vi "Main.vi"() -> ()   [LabVIEW 2020]
uses:
  <vilib>/Modbus/master/Modbus Master.lvclass
  ctl/StationAction.ctl
  <vilib>/Analysis/baseanly.llb/Mean (DBL).vi
  <vilib>/Modbus/master/Create Master Instance (TCP).vi
  <vilib>/Utility/file.llb/Read Delimited Spreadsheet (string).vi
  <vilib>/Analysis/NI_AALBase.lvlib
panel:
  out "原始表格":string[][](table)
  in  "LabVIEW._Application 6":refnum<k7>
  out "权限out":i32
  out "用户名out":string
  out "用户信息out":string[][](array[string]) caption="所有行"
  out "error out 3":errorcluster caption="错误输出"
  out "error out 2":errorcluster caption="错误输出"
  out "error out":errorcluster caption="错误输出"
  out "PLC状态显示":string
  out "PLC_Hd":refnum<class "Modbus Master.lvclass"> caption="TCP主设备实例"
  in  "确定按钮 2":bool
  in  "确定按钮":bool
  in  "LabVIEW._Application 5":refnum<k7>
  out "Cpk原始数据":string[][](array[string])
  in  "Btn_Exit":bool
  in  "选项卡控件":enum32{"工位1", "工位2", "数据分析"}(tab)
  in  "启动信号":u16
  in  "数组":string[](array[string])
  out "工位1_实时压力_Ind":string caption="实时压力"
  out "工位1_数据图表显示":cluster{i32[], dbl[]}[](graph)
  out "工位1_产品型号":string caption="产品型号"
  in  "数组 2":string[](array[string])
  in  "启动信号 2":u16
  out "工位2_产品型号":string caption="产品型号"
  out "工位2_实时压力_Ind":string caption="实时压力"
  out "工位2_数据图表显示":cluster{i32[], dbl[]}[](graph)
  in  "Btn_导出数据":bool
  in  "Btn_保存报告":bool
  out "Cpk":dbl format="%.2f"
  out "均值":dbl
  out "下限值":dbl
  out "上限值":dbl
  out "最小值":dbl
  out "最大值":dbl
  in  "Btn_分析计算":bool
  in  "终止行":u32=10 min=2 step=1
  in  "Cpk保存路径":path
  out "表格控件":string[][](table)
  in  "起始行":u32=1 min=1 step=1
  in  "工位号":enum16{"工位1", "工位2"}(ring)
  out "paramVals":variant
  in  "LabVIEW._Application 4":refnum<k7>
  out "工位1_数据表显示":string[][](table)
  out "bExit?":bool
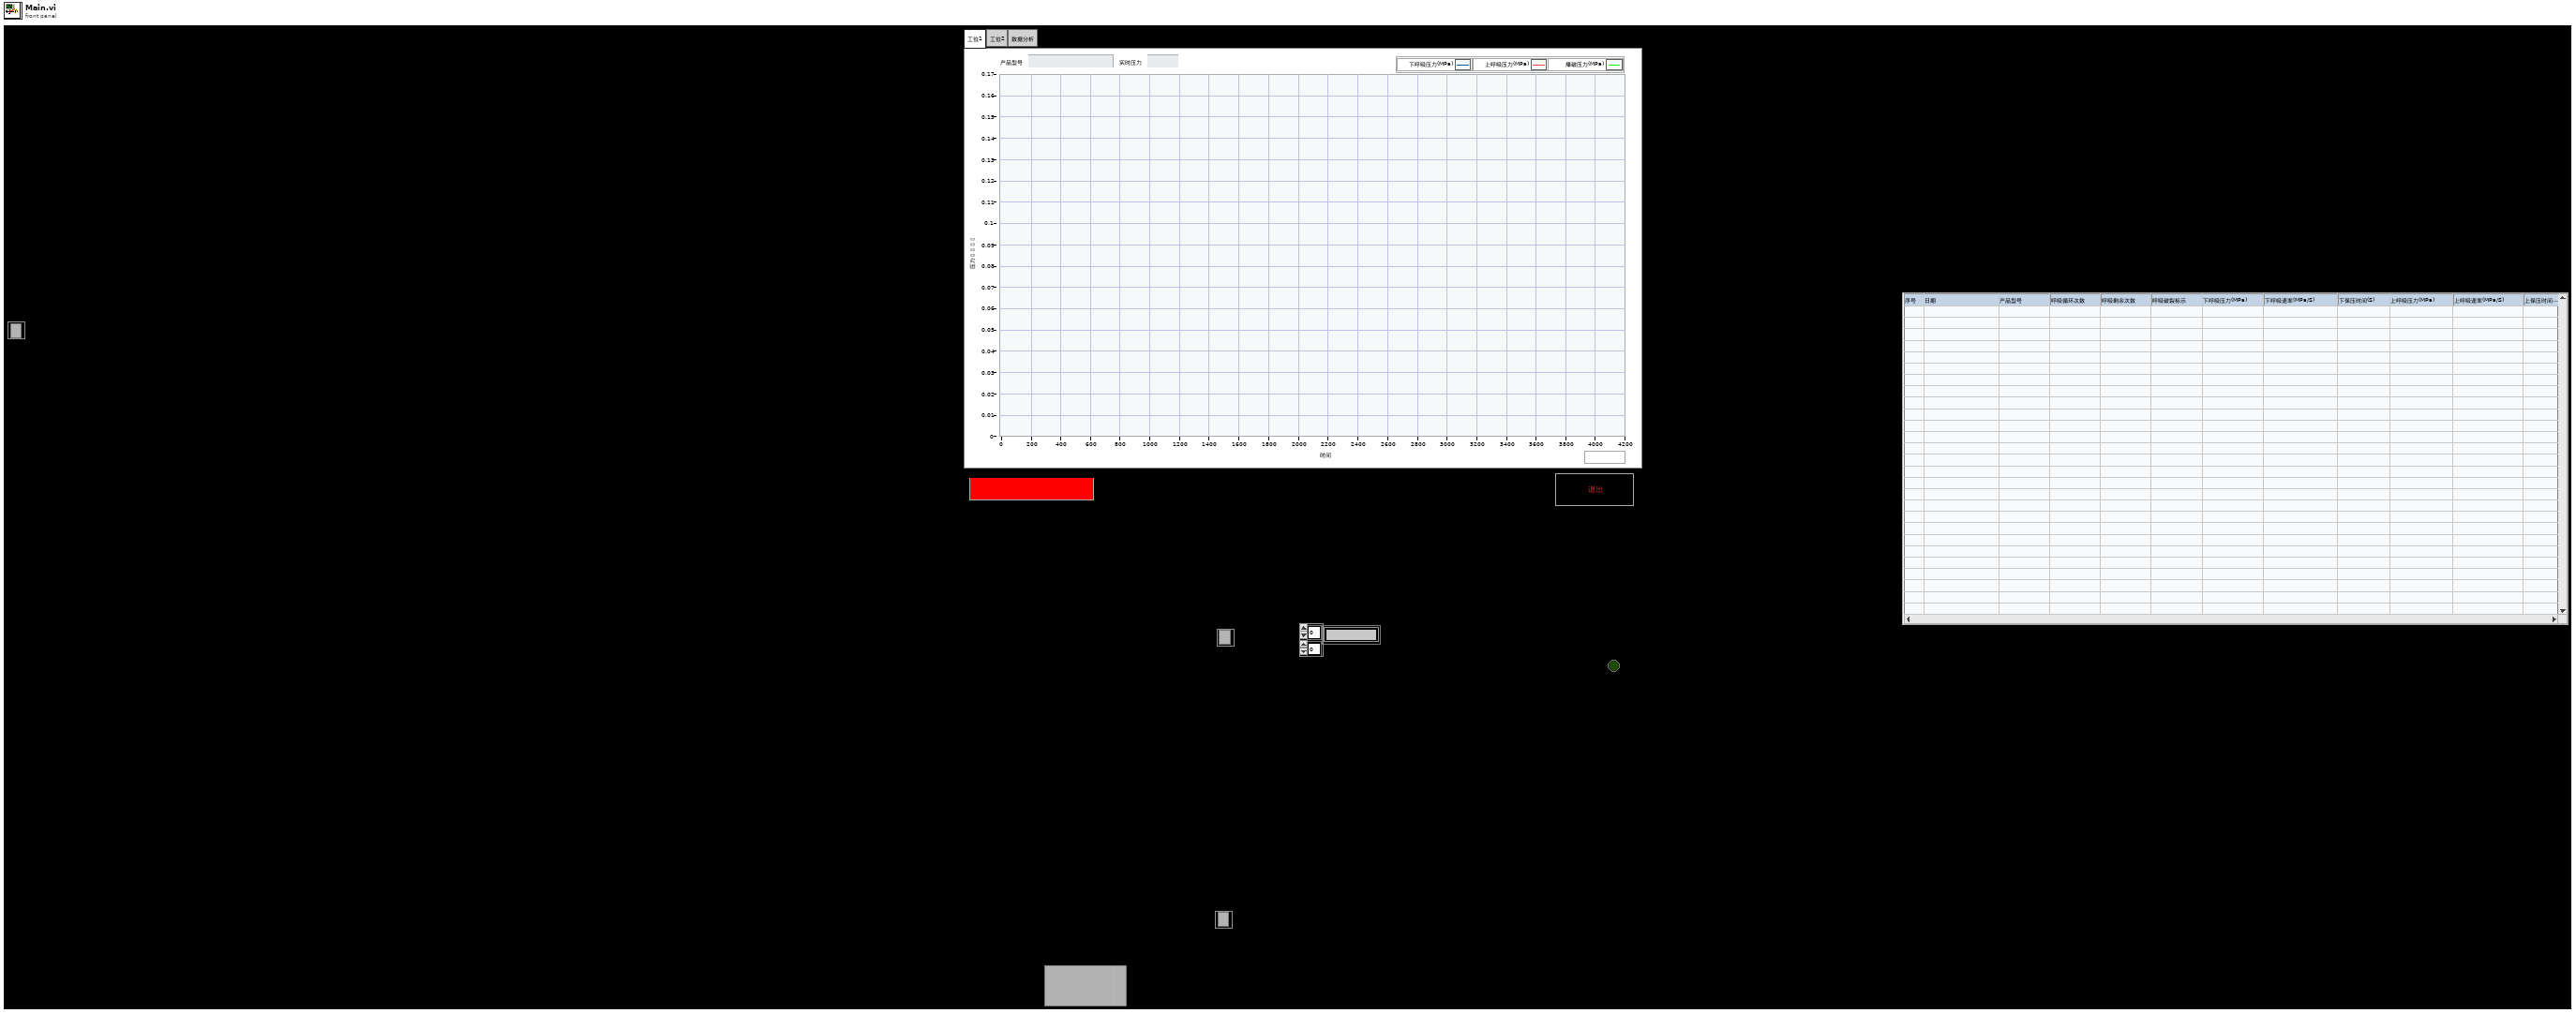
[diagram p1: front panel]
types:
  T1 = typedef "StationAction.ctl" = enum16{"Init", "Monitor", "Done", "Exit"}
  T2 = enum8{"Enabled", "Disabled", "Disabled and Grayed Out"}
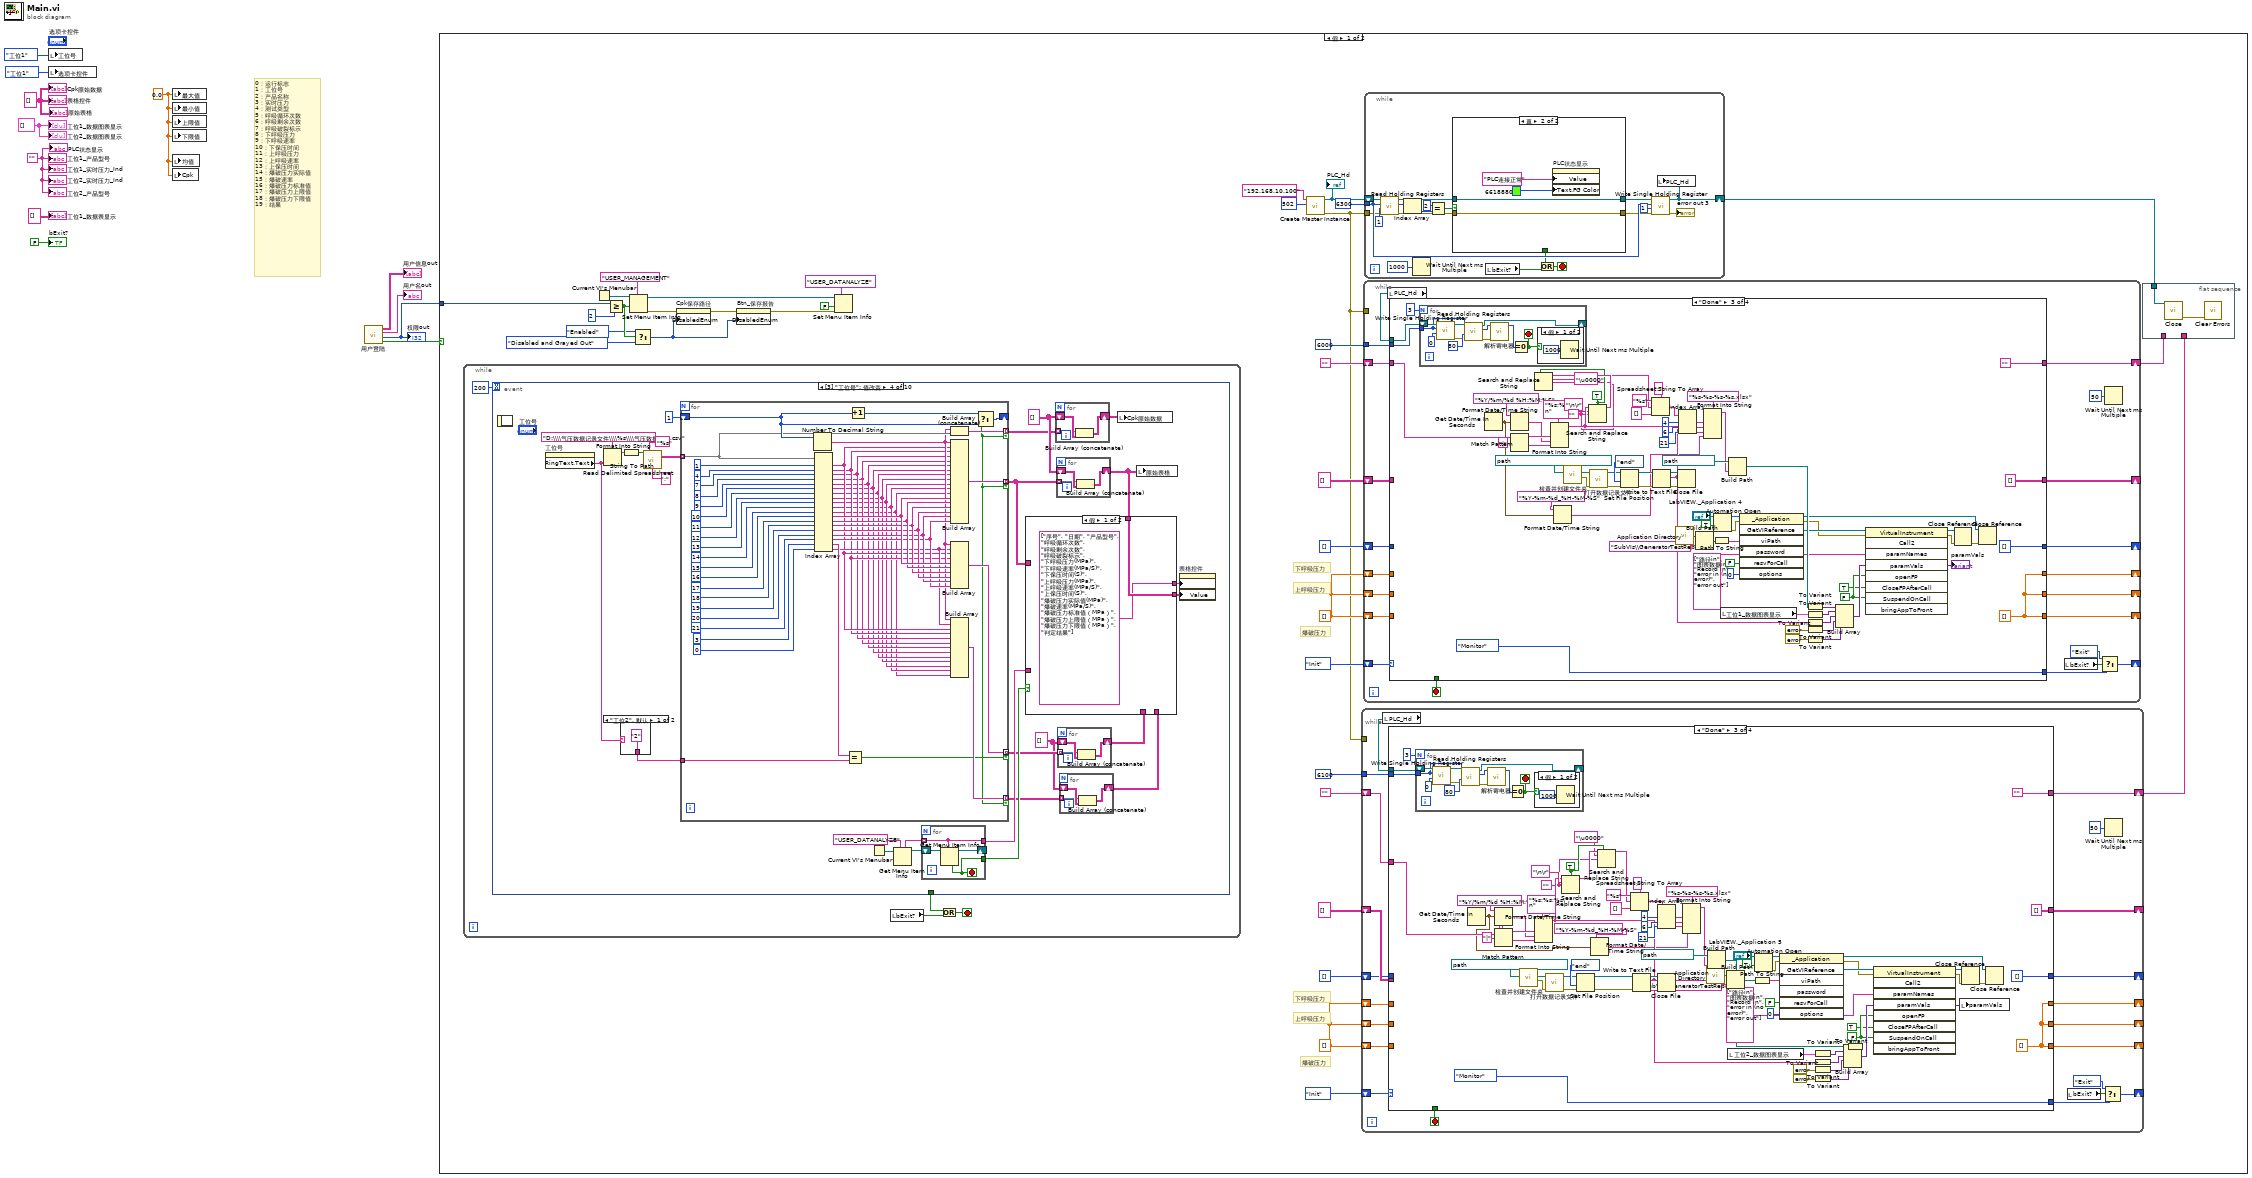
[diagram p0: block diagram]
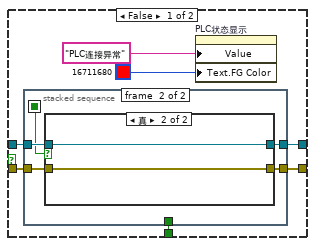
[diagram p2: hidden frame]
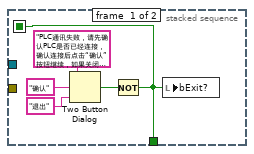
[diagram p3: hidden frame]
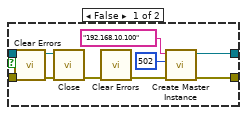
[diagram p4: hidden frame]
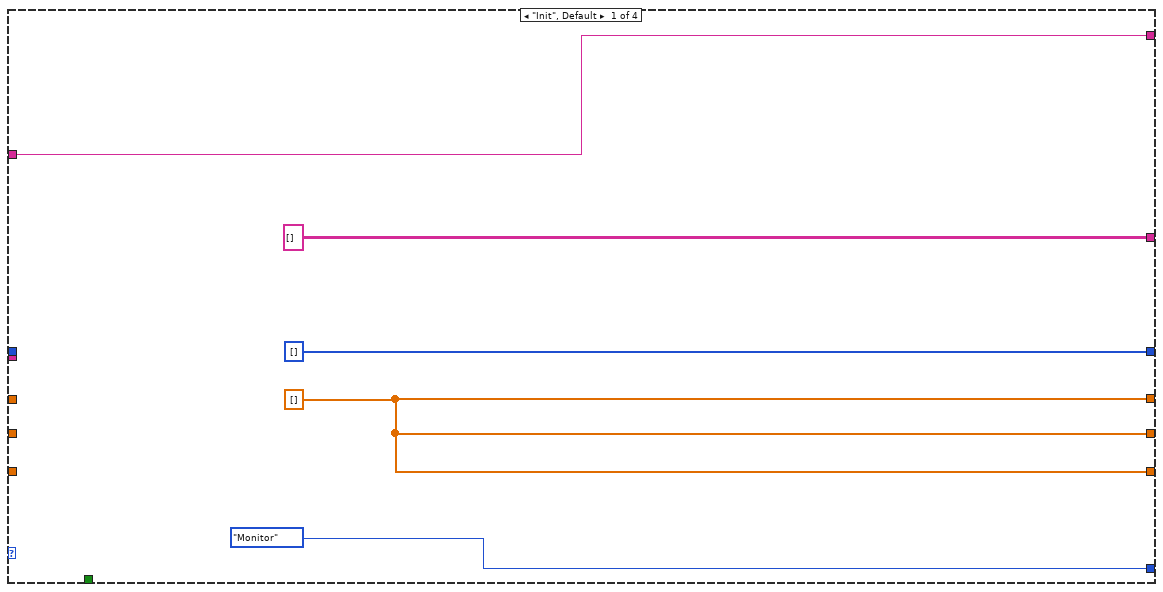
[diagram p5: hidden frame]
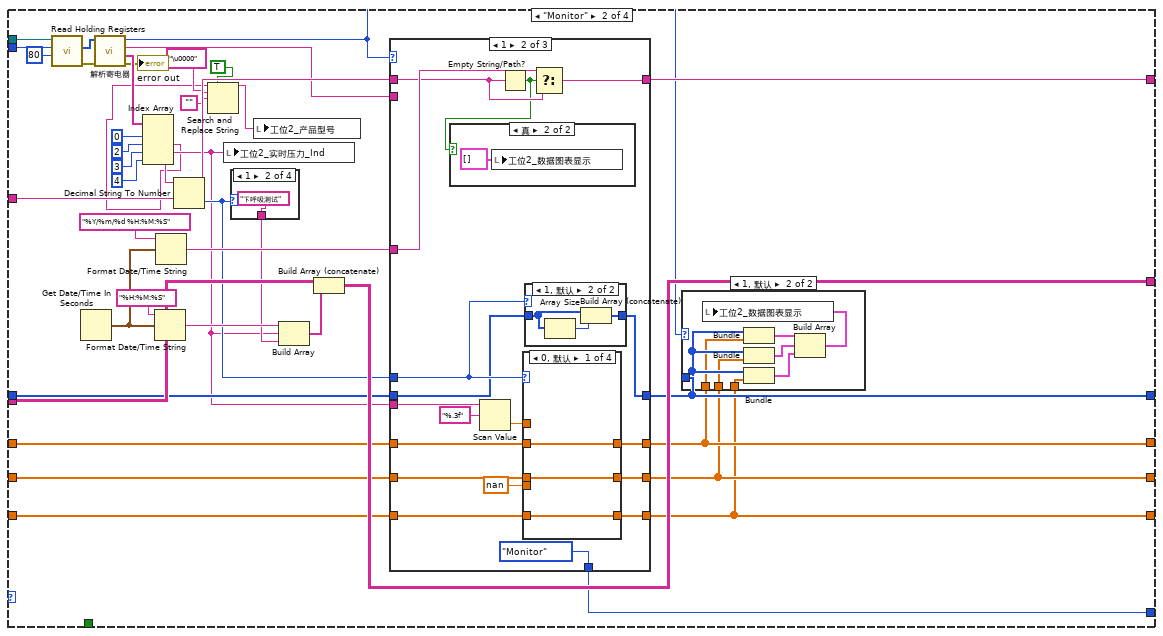
[diagram p6: hidden frame]
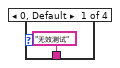
[diagram p8: hidden frame]
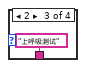
[diagram p9: hidden frame]
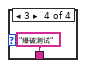
[diagram p10: hidden frame]
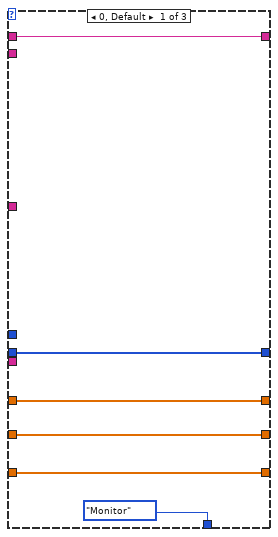
[diagram p11: hidden frame]
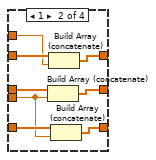
[diagram p14: hidden frame]
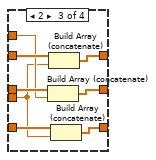
[diagram p15: hidden frame]
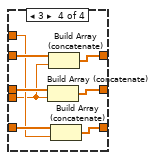
[diagram p16: hidden frame]
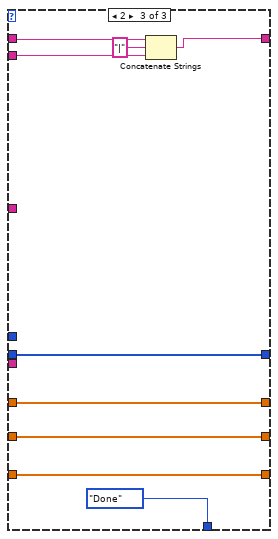
[diagram p17: hidden frame]
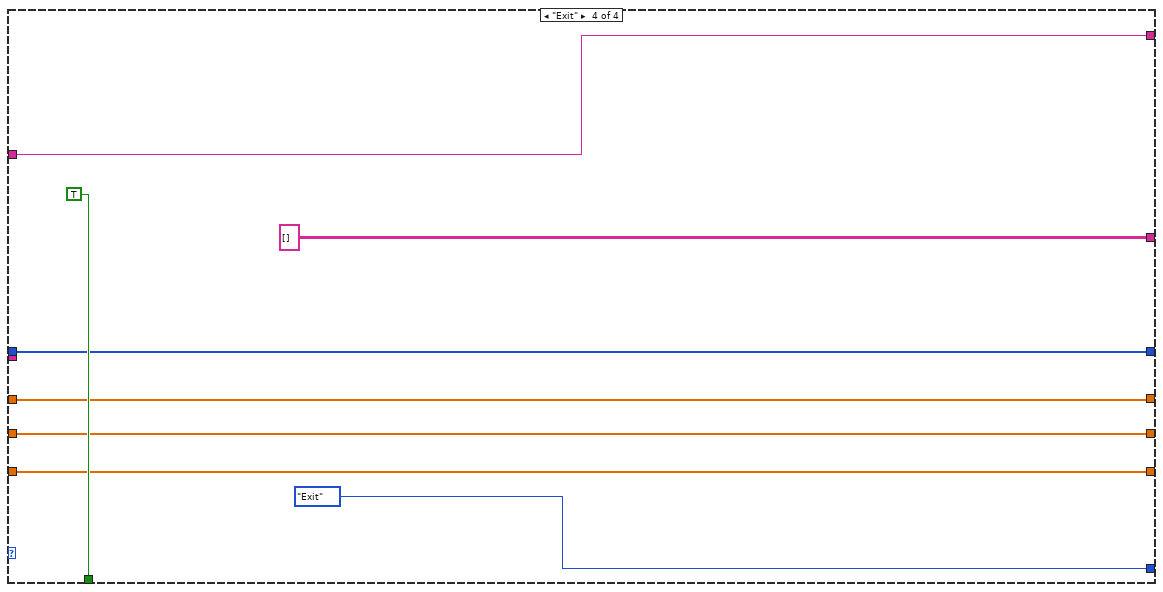
[diagram p19: hidden frame]
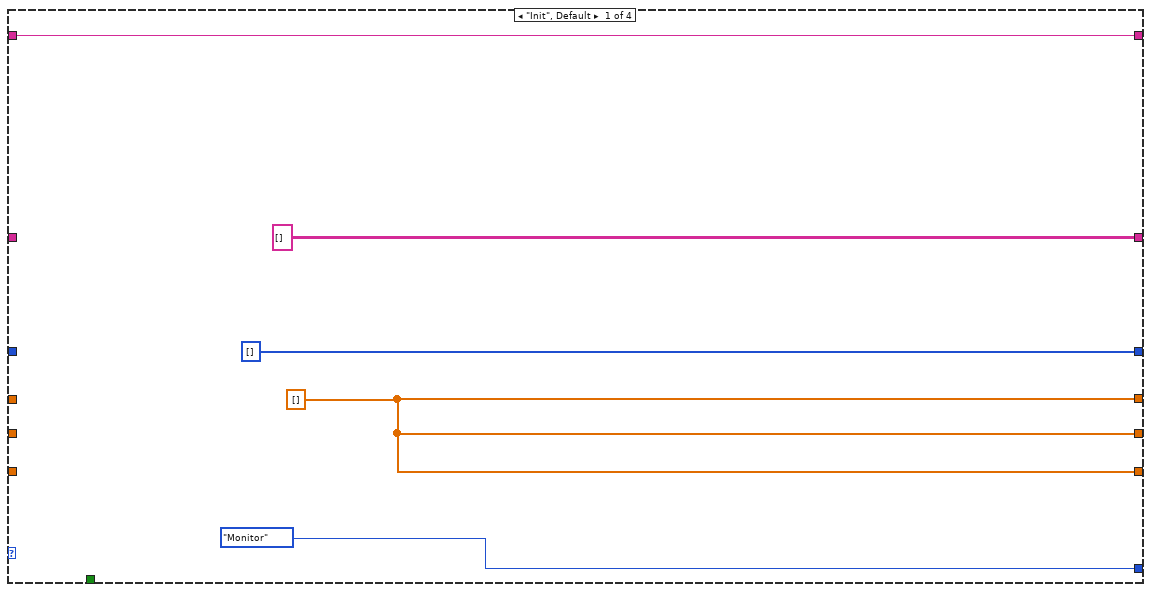
[diagram p20: hidden frame]
diagram:
  w7 = 0.0 ("最大值")
  w1 = string[][] [] ("表格控件")
  w8 = cluster{i32[], dbl[]}[] [] ("添加的数组")
  w6 = ""
  # "0：运行标志\n1：工位号\n2：产品名称\n3：实时压力\n4：测试类型\n5：呼吸循环次数\n6：呼吸剩余次数\n7：呼吸破裂标示\n8：下呼吸压力\n9：下呼吸速率\n10：下保压时间\n11：上呼吸压力\n12：上呼吸速率\n13：上保压时间\n14：爆破压力实际值\n15：爆破速率\n16：爆破压力标准值\n17：爆破压力上限值\n18：爆破压力下限值\n19：结果"
  n1 = local write "工位号"(enum16{"工位1", "工位2"}."工位1" ("工位号")) -> ()
  n2 = local write "选项卡控件"(enum32{"工位1", "工位2", "数据分析"}."工位1" ("选项卡控件")) -> ()
  n3 = local write "最大值"(w7) -> ()
  n4 = local write "最小值"(w7) -> ()
  n5 = local write "上限值"(w7) -> ()
  n6 = local write "下限值"(w7) -> ()
  n7 = local write "均值"(w7) -> ()
  n8 = local write "Cpk"(w7) -> ()
  n9 = call "用户登陆.vi"() -> ("退出"=w5:bool, "权限out"=w2:i32, "用户名out"=→"用户名out":string, "用户信息out"=→"用户信息out":string[][])  [unwired: 8 in]
  "权限out" <- w2
  n10 = case shown="假" w5 {
    tunnel: w2 -> [w44 _]
    frame False {
      w27 = dbl[] []
      w28 = dbl[] []
      # "爆破压力"
      # "上呼吸压力"
      # "下呼吸压力"
      # "爆破压力"
      # "上呼吸压力"
      # "下呼吸压力"
      n11 = while {
        stop <- w585 stop-if-true
        n12 = event shown="[3] \"工位号\": 值改变" {
          selector: _ -> [_ _ _ _ _ _ _ _ _ _]
          dyn-events: _ -> [_ _ _ _ _ _ _ _ _ _]
          timeout: 200 -> [_ _ _ _ _ _ _ _ _ _]
          tunnel: [_ "Btn_Exit" _ _ _ _ _ _ _ _] -> w586
          event Timeout {
            n13 = event-data() -> ()  [unwired: 1 in, 3 out]
          }
          event "Btn_Exit": Value Change {
            n14 = event-data() -> ()  [unwired: 1 in, 1 out]
            n15 = local write "bExit?"("Btn_Exit") -> ()
          }
          event "Btn_分析计算": Value Change {
            n16 = event-data() -> ()  [unwired: 1 in, 1 out]
            n17 = local read "原始表格"() -> (w591:string[][])
            n18 = Subtract(x="终止行", y="起始行") -> (x-y=w593:u32)
            n19 = Less Than 0?(x=w593) -> (x < 0?=w594:bool)
            n20 = Empty Array?(array=w591) -> (empty?=w592:bool)
            n21 = Increment(x=w593) -> (x+1=w589:u32)
            n22 = case shown="假" w592 {
              tunnel: w594 -> [w599 _]
              tunnel: w589 -> [w598 _]
              tunnel: w591 -> [w597 _]
              tunnel: "起始行" -> [w596 _]
              frame False {
                n23 = case shown="假" w599 {
                  tunnel: w598 -> [w601 _]
                  tunnel: w597 -> [w604 _]
                  tunnel: w596 -> [w603 _]
                  frame False {
                    n24 = Greater Or Equal?(x=w601, y=2 ("禁用的索引 (列)")) -> (x >= y?=w602:bool)
                    n25 = case shown="真" w602 {
                      tunnel: w604 -> [_ w634]
                      tunnel: w601 -> [_ w606]
                      tunnel: w603 -> [_ w608]
                      frame False {
                        n26 = One Button Dialog(message="选择数据的数量至少需要2个" ("消息")) -> ()  [unwired: 1 in, 1 out]
                      }
                      frame True {
                        w626 = 0 ("禁用的索引 (列)")
                        n27 = Decrement(x=w608) -> (x-1=w607:u32)
                        n28 = Array Subset(array=w634, index (row)=w607, length (row)=w606) -> (w633:string[][])  [unwired: 2 in]
                        n29 = Fract/Exp String To Number(string=w633) -> (number=w632:dbl[][])  [unwired: 3 in, 1 out]
                        n30 = Index Array(array=w632, index (col) #1=12 ("禁用的索引 (列)"), index (row) #2=w626, index (col) #2=14 ("禁用的索引 (列)"), index (row) #3=w626, index (col) #3=15 ("禁用的索引 (列)"), index (row) #4=w626, index (col) #4=16 ("禁用的索引 (列)")) -> (element #1=w624:dbl[], element #2=w623:dbl, element #3=w620:dbl, element #4=w619:dbl)  [unwired: 1 in]
                        "上限值" <- w620
                        "下限值" <- w619
                        n31 = Array Max & Min(array=w624) -> (max value=→"最大值":dbl, min value=→"最小值":dbl)  [unwired: 2 out]
                        n32 = call-poly <vilib>:"Mean.vi"("X"=w624) -> ("mean"=w622:dbl)  [unwired: 1 out]
                        "均值" <- w622
                        n33 = call <vilib>:"Std Deviation and Variance.vi"("X"=w624) -> ("standard deviation"=w615:dbl)  [unwired: 1 in, 2 out]
                        n34 = Subtract(x=w622, y=w623) -> (x-y=w621:dbl)
                        n35 = Subtract(x=w620, y=w619) -> (x-y=w613:dbl)
                        n36 = Absolute Value(x=w621) -> (abs(x)=w618:dbl)
                        n37 = Multiply(x=w615, y=3.0) -> (x*y=w617:dbl)
                        n38 = Multiply(x=w615, y=6.0) -> (x*y=w612:dbl)
                        n39 = Divide(x=w618, y=w617) -> (x/y=w610:dbl)
                        n40 = Divide(x=w613, y=w612) -> (x/y=w611:dbl)
                        n41 = Subtract(x=w611, y=w610) -> (x-y=→"Cpk":dbl)
                      }
                    }
                  }
                  frame True {
                    n42 = One Button Dialog(message="终止行必须大于起始行" ("消息")) -> ()  [unwired: 1 in, 1 out]
                  }
                }
              }
              frame True {
                n43 = One Button Dialog(message="参与计算Cpk的数据不可以为空" ("消息")) -> ()  [unwired: 1 in, 1 out]
              }
            }
          }
          event "工位号": Value Change {
            w639 = string[][] []
            w654 = string[][] []
            n44 = event-data() -> ()  [unwired: 1 in, 1 out]
            n45 = property on="工位号" class="Enum (严格)"() -> ("RingText.Text"=w657:string)  [unwired: 2 in, 2 out]
            n46 = Format Into String(format string="D:\\\\气压数据记录文件\\\\%s\\\\气压数据记录.csv" ("格式字符串"), w657) -> (resulting string=w661:string)  [unwired: 2 in, 1 out]
            n47 = case shown="\"工位2\", 默认" w657 {
              tunnel: ["2" ("delimiter (\\t)") "1" ("delimiter (\\t)")] -> w656
              frame "工位2", Default {
              }
              frame "工位1" {
              }
            }
            n48 = String To Path(string=w661) -> (path=w660:path)
            n49 = call-poly <vilib>:"Read Delimited Spreadsheet.vi"("file path (dialog if empty)"=w660, "format (%s)"="%s", "delimiter (\\t)"=";" ("delimiter (\\t)")) -> ("all rows"=w658:string[][])  [unwired: 7 in, 5 out]
            n50 = for {
              tunnel: w658 -> [w721] mode=indexing
              tunnel: [w728] -> w645 mode=indexing if=w697
              tunnel: w656 -> [w727]
              tunnel: [w720] -> w653 mode=indexing if=w697
              shift-right: [w723] -> _
              shift-left: 1 -> [w722]
              tunnel: [w712] -> w641 mode=indexing if=w697
              tunnel: [w698] -> w638 mode=indexing if=w697
              n51 = Number To Decimal String(number=w722) -> (decimal integer string=w711:string)  [unwired: 1 in]
              n52 = Index Array(array=w721, index #1=1 ("索引"), index #2=4 ("索引"), index #3=7 ("索引"), index #4=8 ("索引"), index #5=9 ("索引"), index #6=10 ("索引"), index #7=11 ("索引"), index #8=12 ("索引"), index #9=13 ("索引"), index #10=14 ("索引"), index #11=15 ("索引"), index #12=16 ("索引"), index #13=17 ("索引"), index #14=18 ("索引"), index #15=19 ("索引"), index #16=20 ("索引"), index #17=21 ("索引"), index #18=3 ("索引"), index #19=0 ("索引")) -> (element #1=w709:string, element #2=w708:string, element #3=w707:string, element #4=w706:string, element #5=w705:string, element #6=w704:string, element #7=w703:string, element #8=w702:string, element #9=w701:string, element #10=w700:string, element #11=w699:string, element #12=w718:string, element #13=w717:string, element #14=w716:string, element #15=w715:string, element #16=w714:string, element #17=w713:string, element #18=w725:string, element #19=w710:string)
              n53 = Equal?(x=w725, y=w727) -> (x = y?=w697:bool)
              n54 = Increment(x=w722) -> (x+1=w724:i32)
              n55 = Build Array (concatenate)(w711, w721) -> (w720:string[])
              n56 = Build Array(w711, w709, w708, w707, w706, w705, w704, w703, w702, w701, w700, w699, w718, w717, w716, w715, w714, w713) -> (w728:string[])
              n57 = Build Array(w711, w710, w709, w708, w718, w717, w716, w715, w714, w713) -> (w712:string[])
              n58 = Build Array(w711, w710, w709, w708, w707, w706, w705, w704, w703, w702, w701, w700, w699) -> (w698:string[])
              n59 = Select(t=w724, s=w697, f=w722) -> (s? t:f=w723:i32)
            }
            n60 = Current VI's Menubar() -> (w651:refnum<k9>)
            n61 = Get Menu Item Info(7:"USER_DATANALYZE" ("项标识符"), 11:w651) -> (3:w648:refnum<k9>, 5:w649:string[])  [unwired: 1 in, 5 out]
            n62 = for {
              tunnel: w649 -> [w686] mode=indexing
              shift-right: [w687] -> _
              shift-left: w648 -> [w688]
              tunnel: [w686] -> w646
              tunnel: [w685] -> w647
              stop <- w685 stop-if-true
              n63 = Get Menu Item Info(7:w686, 11:w688) -> (3:w687:refnum<k9>, 4:w685:bool)  [unwired: 1 in, 5 out]
            }
            n64 = for {
              shift-right: [w693] -> w652
              shift-left: w654 -> [w694]
              tunnel: w653 -> [w692] mode=indexing
              n65 = Build Array (concatenate)(w692, w694) -> (w693:string[][])
            }
            n66 = for {
              shift-right: [w690] -> w644
              shift-left: w654 -> [w691]
              tunnel: w645 -> [w689] mode=indexing
              n67 = Build Array (concatenate)(w689, w691) -> (w690:string[][])
            }
            n68 = for {
              shift-right: [w668] -> w640
              shift-left: w639 -> [w669]
              tunnel: w641 -> [w667] mode=indexing
              n69 = Build Array (concatenate)(w667, w669) -> (w668:string[][])
            }
            n70 = for {
              shift-right: [w665] -> w637
              shift-left: w639 -> [w666]
              tunnel: w638 -> [w664] mode=indexing
              n71 = Build Array (concatenate)(w664, w666) -> (w665:string[][])
            }
            n72 = case shown="假" w647 {
              tunnel: w646 -> [_ w677]
              tunnel: w645 -> [_ w678]
              tunnel: [w671 w675] -> w643
              tunnel: w644 -> [w671 w676]
              tunnel: [string[] ["序号", "日期", "产品型号", "呼吸循环次数", "呼吸剩余次数", "呼吸破裂标示", "下呼吸压力(MPa)", "下呼吸速率(MPa/S)", "下保压时间(S)", "上呼吸压力(MPa)", "上呼吸速率(MPa/S)", "上保压时间(S)", "爆破压力实际值(MPa)", "爆破速率(MPa/S)", "爆破压力标准值（MPa）", "爆破压力上限值（MPa）", "爆破压力下限值（MPa）", "判定结果"] w674] -> w642
              tunnel: w640 -> [_ w673]
              tunnel: w637 -> [_ w672]
              frame False {
              }
              frame True {
                n73 = case shown="\"假\", 默认" w677 {
                  tunnel: w678 -> [_ _ _]
                  tunnel: w676 -> [w680 _ _]
                  tunnel: [w680 w681 w683] -> w675
                  tunnel: [string[] ["序号", "日期", "产品型号", "呼吸循环次数", "呼吸剩余次数", "呼吸破裂标示", "下呼吸压力(MPa)", "下呼吸速率(MPa/S)", "下保压时间(S)", "上呼吸压力(MPa)", "上呼吸速率(MPa/S)", "上保压时间(S)", "爆破压力实际值(MPa)", "爆破速率(MPa/S)", "爆破压力标准值（MPa）", "爆破压力上限值（MPa）", "爆破压力下限值（MPa）", "判定结果"] w682 w684] -> w674
                  tunnel: w673 -> [_ w681 _]
                  tunnel: w672 -> [_ _ w683]
                  frame "假", Default {
                  }
                  frame "USER_BLASTING_REC" {
                    w682 = string[] ["序号", "开始时间", "结束时间", "产品型号", "爆破压力实际值(MPa)", "爆破速率(MPa/S)", "爆破压力标准值（MPa）", "爆破压力上限值（MPa）", "爆破压力下限值（MPa）", "判定结果"]  # 爆破记录
                  }
                  frame "USER_BREATHE_REC" {
                    w684 = string[] ["序号", "开始时间", "结束时间", "产品型号", "呼吸循环次数", "呼吸剩余次数", "呼吸破裂标示", "下呼吸压力(MPa)", "下呼吸速率(MPa/S)", "下保压时间(S)", "上呼吸压力(MPa)", "上呼吸速率(MPa/S)", "上保压时间(S)"]  # 呼吸记录
                  }
                }
              }
            }
            n74 = local write "Cpk原始数据"(w652) -> ()
            n75 = local write "原始表格"(w644) -> ()
            n76 = property on="表格控件" class="Tbl (严格)"("Column Headers[]"=w642, "Value"=w643) -> ()  [unwired: 2 in, 2 out]
          }
          event "选项卡控件": Value Change {
            # "0：开始时间\n1：结束时间\n2：运行标志\n3：工位号\n4：产品名称\n5：实时压力\n6：测试类型\n7：呼吸循环次数\n8：呼吸剩余次数\n9：呼吸破裂标示\n10：下呼吸压力\n11：下呼吸速率\n12：下保压时间\n13：上呼吸压力\n14：上呼吸速率\n15：上保压时间\n16：爆破压力实际值\n17：爆破速率\n18：爆破压力标准值\n19：爆破压力上限值\n20：爆破压力下限值\n21：结果"
            n77 = event-data() -> ("NewVal"=w746:enum32{"工位1", "工位2", "数据分析"})  [unwired: 1 in]
            n78 = case shown="\"数据分析\"" w746 {
              frame "工位1", Default {
                n79 = Current VI's Menubar() -> (w747:refnum<k9>)
                n80 = Set Menu Item Info(7:"USER_DATANALYZE" ("项标识符"), 9:FALSE ("已启用"), 11:w747) -> ()  [unwired: 4 in, 2 out]
              }
              frame "数据分析" {
                w750 = FALSE
                w759 = TRUE ("已启用")
                w768 = string[][] []
                n81 = property on="工位号" class="Enum (严格)"() -> ("RingText.Text"=w772:string)  [unwired: 2 in, 2 out]
                n82 = Format Into String(format string="D:\\\\气压数据记录文件\\\\%s\\\\气压数据记录.csv" ("格式字符串"), w772) -> (resulting string=w779:string)  [unwired: 2 in, 1 out]
                n83 = String To Path(string=w779) -> (path=w778:path)
                n84 = case shown="\"工位2\", 默认" w772 {
                  tunnel: ["2" ("delimiter (\\t)") "1" ("delimiter (\\t)")] -> w771
                  frame "工位2", Default {
                  }
                  frame "工位1" {
                  }
                }
                n85 = call-poly <vilib>:"Read Delimited Spreadsheet.vi"("file path (dialog if empty)"=w778, "format (%s)"="%s", "delimiter (\\t)"=";" ("delimiter (\\t)")) -> ("all rows"=w774:string[][])  [unwired: 7 in, 5 out]
                n86 = for {
                  tunnel: w774 -> [w788] mode=indexing
                  tunnel: [w801] -> w767 mode=indexing if=w797
                  tunnel: w771 -> [w799]
                  tunnel: [w790] -> w770 mode=indexing if=w797
                  shift-right: [w795] -> _
                  shift-left: 1 -> [w793]
                  n87 = Number To Decimal String(number=w793) -> (decimal integer string=w789:string)  [unwired: 1 in]
                  n88 = Build Array (concatenate)(w789, w788) -> (w790:string[])
                  n89 = Index Array(array=w788, index #1=1 ("索引"), index #2=4 ("索引"), index #3=7 ("索引"), index #4=8 ("索引"), index #5=9 ("索引"), index #6=10 ("索引"), index #7=11 ("索引"), index #8=12 ("索引"), index #9=13 ("索引"), index #10=14 ("索引"), index #11=15 ("索引"), index #12=16 ("索引"), index #13=17 ("索引"), index #14=18 ("索引"), index #15=19 ("索引"), index #16=20 ("索引"), index #17=21 ("索引"), index #18=3 ("索引")) -> (element #1=w815:string, element #2=w796:string, element #3=w798:string, element #4=w814:string, element #5=w813:string, element #6=w812:string, element #7=w811:string, element #8=w810:string, element #9=w809:string, element #10=w808:string, element #11=w807:string, element #12=w800:string, element #13=w806:string, element #14=w805:string, element #15=w804:string, element #16=w803:string, element #17=w802:string, element #18=w791:string)
                  n90 = Equal?(x=w791, y=w799) -> (x = y?=w797:bool)
                  n91 = Increment(x=w793) -> (x+1=w794:i32)
                  n92 = Build Array(w789, w815, w796, w798, w814, w813, w812, w811, w810, w809, w808, w807, w800, w806, w805, w804, w803, w802) -> (w801:string[])
                  n93 = Select(t=w794, s=w797, f=w793) -> (s? t:f=w795:i32)
                }
                n94 = Current VI's Menubar() -> (w765:refnum<k9>)
                n95 = Set Menu Item Info(7:"USER_DATANALYZE" ("项标识符"), 9:TRUE ("已启用"), 11:w765) -> (0:w760:errorcluster, 3:w763:refnum<k9>)  [unwired: 4 in]
                n96 = Set Menu Item Info(6:w759, 7:"USER_DATA_ALL" ("项标识符"), 8:w760, 9:w759, 11:w763) -> (0:w755:errorcluster, 3:w756:refnum<k9>)  [unwired: 2 in]
                n97 = Set Menu Item Info(6:w750, 7:"USER_BLASTING_REC" ("项标识符"), 8:w755, 9:TRUE ("已启用"), 11:w756) -> (0:w751:errorcluster, 3:w752:refnum<k9>)  [unwired: 2 in]
                n98 = Set Menu Item Info(6:w750, 7:"USER_BREATHE_REC" ("项标识符"), 8:w751, 9:TRUE ("已启用"), 11:w752) -> ()  [unwired: 2 in, 2 out]
                n99 = for {
                  shift-right: [w781] -> w764
                  shift-left: w768 -> [w782]
                  tunnel: w767 -> [w780] mode=indexing
                  n100 = Build Array (concatenate)(w780, w782) -> (w781:string[][])
                }
                n101 = for {
                  shift-right: [w784] -> w769
                  shift-left: w768 -> [w785]
                  tunnel: w770 -> [w783] mode=indexing
                  n102 = Build Array (concatenate)(w783, w785) -> (w784:string[][])
                }
                n103 = local write "Cpk原始数据"(w769) -> ()
                n104 = local write "表格控件"(w764) -> ()
                n105 = local write "原始表格"(w764) -> ()
              }
            }
          }
          event "Btn_保存报告": Value Change {
            n106 = event-data() -> ()  [unwired: 1 in, 1 out]
            n107 = local read "起始行"() -> (w835:u32)
            n108 = local read "终止行"() -> (w833:u32)
            n109 = Subtract(x=w833, y=w835) -> (x-y=w836:u32)
            n110 = Increment(x=w836) -> (x+1=w834:u32)
            n111 = Less Than 0?(x=w836) -> (x < 0?=w837:bool)
            n112 = case shown="假" w837 {
              tunnel: w834 -> [w839 _]
              tunnel: w835 -> [w842 _]
              tunnel: w833 -> [w841 _]
              frame False {
                n113 = Greater Or Equal?(x=w839, y=2 ("options")) -> (x >= y?=w840:bool)
                n114 = case shown="真" w840 {
                  tunnel: w842 -> [_ w846]
                  tunnel: w839 -> [_ w845]
                  tunnel: w841 -> [_ w844]
                  frame False {
                    n115 = One Button Dialog(message="选择数据的数量必须为10个" ("消息")) -> ()  [unwired: 1 in, 1 out]
                  }
                  frame True {
                    n116 = local read "Cpk原始数据"() -> (w847:string[][])
                    n117 = Empty String/Path?(string/path="Cpk保存路径") -> (empty?=w850:bool)
                    n118 = Empty Array?(array=w847) -> (empty?=w848:bool)
                    n119 = Or(x=w850, y=w848) -> (x .or. y?=w849:bool)
                    n120 = case shown="假" w849 {
                      tunnel: "Cpk保存路径" -> [w861 _]
                      tunnel: w847 -> [w860 _]
                      tunnel: w846 -> [w857 _]
                      tunnel: w845 -> [w859 _]
                      tunnel: w844 -> [w858 _]
                      frame False {
                        n121 = Decrement(x=w857) -> (x-1=w854:u32)
                        n122 = Array Subset(array=w860, index (row)=w854, length (row)=w859) -> (w853:string[][])  [unwired: 2 in]
                        n123 = Number To Decimal String(number=w857) -> (decimal integer string=w856:string)  [unwired: 1 in]
                        n124 = Number To Decimal String(number=w858) -> (decimal integer string=w855:string)  [unwired: 1 in]
                        n125 = Empty Array?(array=w853) -> (empty?=w852:bool)
                        n126 = case shown="假" w852 {
                          tunnel: w861 -> [w865 _]
                          tunnel: w856 -> [w864 _]
                          tunnel: w855 -> [w863 _]
                          tunnel: w853 -> [w862 _]
                          frame False {
                            n127 = disable-structure shown="启用" {
                              disable-tunnel: w865 -> [w875 w899]
                              disable-tunnel: w864 -> [w874 w901]
                              disable-tunnel: w863 -> [w873 w900]
                              disable-tunnel: w862 -> [w870 w902]
                              frame Enabled {
                                w880 = FALSE ("CloseFPAfterCall")
                                n128 = local read "LabVIEW._Application 4"() -> (w898:refnum<k7>)
                                n129 = call <vilib>:"Application Directory.vi"() -> ("Application Directory"=w869:path)
                                n130 = Build Path(base path=w869, name or relative path="SubVIs\\GeneratorCpkReport.vi") -> (appended path=w867:path)
                                n131 = Path To String(path=w867) -> (string=w866:string)
                                n132 = Automation Open(Automation Refnum=w898, 9:TRUE ("open new instance (false)")) -> (Automation Refnum=w891:refnum<k7>, error out=w890:errorcluster)  [unwired: 2 in]
                                n133 = invoke class="_Application" method="GetVIReference"(reference=w891, error in=w890, "viPath"=w866, "resvForCall"=FALSE, "options"=0) -> (reference out=w884:refnum<k7>, error out=w888:errorcluster, "GetVIReference"=w889:refnum<k7>)  [unwired: 2 in, 4 out]
                                n134 = To Variant(anything=w875) -> (Variant=w892:variant)
                                n135 = To Variant(anything=w870) -> (Variant=w893:variant)
                                n136 = To Variant(anything=errorcluster {"status"=FALSE, "code"=0, "source"=""} ("错误输出")) -> (Variant=w894:variant)
                                n137 = To Variant(anything=errorcluster {"status"=FALSE, "code"=0, "source"=""} ("错误输出")) -> (Variant=w896:variant)
                                n138 = To Variant(anything=w874) -> (Variant=w872:variant)
                                n139 = To Variant(anything=w873) -> (Variant=w871:variant)
                                n140 = Build Array(w892, w893, w894, w896, w872, w871) -> (w895:variant[])
                                n141 = invoke class="VirtualInstrument" method="Call2"(reference=w889, error in=w888, "paramNames"=string[] ["路径in", "测试数据in", "error in (no error)", "error out", "起始行in", "结束行in"], "paramVals"=w895, "openFP"=w880, "CloseFPAfterCall"=TRUE, "SuspendOnCall"=w880) -> (reference out=w887:refnum<k7>, error out=w886:errorcluster, "paramVals"=w897:variant)  [unwired: 2 in, 6 out]
                                n142 = local write "paramVals"(w897) -> ()
                                n143 = Close Reference(reference=w887, error in (no error)=w886) -> (error out=w885:errorcluster)
                                n144 = Close Reference(reference=w884, error in (no error)=w885) -> ()  [unwired: 1 out]
                              }
                              frame Disabled {
                                n145 = call "GeneratorCpkReport.vi"("结束行in"=w900, "起始行in"=w901, "测试数据in"=w902, "路径in"=w899) -> ()  [unwired: 7 in, 1 out]
                              }
                            }
                          }
                          frame True {
                            n146 = One Button Dialog(message="选取的数据不能为空" ("消息")) -> ()  [unwired: 1 in, 1 out]
                          }
                        }
                      }
                      frame True {
                        n147 = One Button Dialog(message="Cpk报文路径和数据表不可以为空" ("消息")) -> ()  [unwired: 1 in, 1 out]
                      }
                    }
                  }
                }
              }
              frame True {
                n148 = One Button Dialog(message="终止行必须大于起始行" ("消息")) -> ()  [unwired: 1 in, 1 out]
              }
            }
          }
          event "Btn_导出数据": Value Change {
            n149 = event-data() -> ()  [unwired: 1 in, 1 out]
            n150 = call "文件对话框"("prompt"="数据导入路径", "pattern (all files)"=".xlsx") -> ("selected path"=w908:path, "cancelled"=w909:bool, "error out"=w907:errorcluster)  [unwired: 10 in, 1 out]
            n151 = case shown="假" w909 {
              tunnel: w908 -> [w915 _]
              tunnel: w907 -> [_ _]
              frame False {
                w925 = "SubVIs\\导出数据.vi"  # SubVIs\导出数据.vi
                w921 = FALSE ("CloseFPAfterCall")
                n152 = property on="表格控件" class="Tbl (严格)"() -> ("Column Headers[]"=w914:string[], "Value"=w913:string[][])  [unwired: 2 in, 2 out]
                n153 = call <vilib>:"Application Directory.vi"() -> ("Application Directory"=w912:path)
                n154 = Build Path(base path=w912, name or relative path=w925) -> (appended path=w941:path)
                n155 = Path To String(path=w941) -> (string=w942:string)
                n156 = Automation Open(Automation Refnum="LabVIEW._Application 6", 9:TRUE ("open new instance (false)")) -> (Automation Refnum=w932:refnum<k7>, error out=w933:errorcluster)  [unwired: 2 in]
                n157 = invoke class="_Application" method="GetVIReference"(reference=w932, error in=w933, "viPath"=w942, "resvForCall"=FALSE, "options"=0) -> (reference out=w939:refnum<k7>, error out=w935:errorcluster, "GetVIReference"=w934:refnum<k7>)  [unwired: 2 in, 4 out]
                n158 = To Variant(anything=w915) -> (Variant=w931:variant)
                n159 = To Variant(anything=w914) -> (Variant=w930:variant)
                n160 = To Variant(anything=errorcluster {"status"=FALSE, "code"=0, "source"=""} ("错误输出")) -> (Variant=w929:variant)
                n161 = To Variant(anything=errorcluster {"status"=FALSE, "code"=0, "source"=""} ("错误输出")) -> (Variant=w927:variant)
                n162 = To Variant(anything=w913) -> (Variant=w940:variant)
                n163 = Build Array(w931, w930, w929, w927, w940) -> (w928:variant[])
                n164 = invoke class="VirtualInstrument" method="Call2"(reference=w934, error in=w935, "paramNames"=string[] ["path", "column headers", "error in (no error)", "error out", "text data"], "paramVals"=w928, "openFP"=w921, "CloseFPAfterCall"=TRUE, "SuspendOnCall"=w921) -> (reference out=w936:refnum<k7>, error out=w937:errorcluster, "paramVals"=w926:variant)  [unwired: 2 in, 6 out]
                n165 = local write "paramVals"(w926) -> ()
                n166 = Close Reference(reference=w936, error in (no error)=w937) -> (error out=w938:errorcluster)
                n167 = Close Reference(reference=w939, error in (no error)=w938) -> (error out=w916:errorcluster)
                n168 = flat-sequence {
                  tunnel: w916 -> [_]
                  frame #0 {
                    n169 = One Button Dialog(message="数据导出完成" ("消息")) -> ()  [unwired: 1 in, 1 out]
                  }
                }
              }
              frame True {
              }
            }
          }
          event Menu Selection (User) {
            n170 = event-data() -> ("ItemTag"=w944:string)  [unwired: 1 in]
            n171 = case shown="\"USER_FILE_ANALYZE\"" w944 {
              frame "假", Default {
              }
              frame "USER_MANAGEMENT" {
                n172 = local read "用户信息out"() -> (w948:string[][])
                n173 = local read "用户名out"() -> (w947:string)
                n174 = local read "权限out"() -> (w946:i32)
                n175 = call "用户管理.vi"("权限"=w946, "用户名"=w947, "用户信息"=w948) -> ("项名"=w945:string[][])  [unwired: 8 in]
                n176 = local write "用户信息out"(w945) -> ()
              }
              frame "USER_FILE_STATION1" {
                n177 = property on="选项卡控件" class="TabCtl (严格)"("Val(Sgnl)"=enum32{"工位1", "工位2", "数据分析"}."工位1" ("值(信号)")) -> ()  [unwired: 2 in, 2 out]
              }
              frame "USER_FILE_STATION2" {
                n178 = property on="选项卡控件" class="TabCtl (严格)"("Val(Sgnl)"=enum32{"工位1", "工位2", "数据分析"}."工位2" ("值(信号)")) -> ()  [unwired: 2 in, 2 out]
              }
              frame "USER_FILE_ANALYZE" {
                n179 = property on="选项卡控件" class="TabCtl (严格)"("Val(Sgnl)"=enum32{"工位1", "工位2", "数据分析"}."数据分析" ("值(信号)")) -> ()  [unwired: 2 in, 2 out]
              }
              frame "USER_DATA_ALL" {
                w952 = FALSE ("已勾选")
                w961 = TRUE ("已启用")
                n180 = Current VI's Menubar() -> (w963:refnum<k9>)
                n181 = Set Menu Item Info(6:w961, 7:"USER_DATA_ALL" ("项标识符"), 9:w961, 11:w963) -> (0:w957:errorcluster, 3:w958:refnum<k9>)  [unwired: 3 in]
                n182 = Set Menu Item Info(6:w952, 7:"USER_BLASTING_REC" ("项标识符"), 8:w957, 9:TRUE ("已启用"), 11:w958) -> (0:w953:errorcluster, 3:w954:refnum<k9>)  [unwired: 2 in]
                n183 = local read "工位号"() -> (w964:enum16{"工位1", "工位2"})
                n184 = property on="工位号" class="Enum (严格)"("Val(Sgnl)"=w964) -> ()  [unwired: 2 in, 2 out]
                n185 = Set Menu Item Info(6:w952, 7:"USER_BREATHE_REC" ("项标识符"), 8:w953, 9:TRUE ("已启用"), 11:w954) -> ()  [unwired: 2 in, 2 out]
              }
              frame "USER_BLASTING_REC" {
                w973 = TRUE ("已启用")
                n186 = Current VI's Menubar() -> (w977:refnum<k9>)
                n187 = Set Menu Item Info(6:FALSE ("已勾选"), 7:"USER_DATA_ALL" ("项标识符"), 9:TRUE ("已启用"), 11:w977) -> (0:w971:errorcluster, 3:w972:refnum<k9>)  [unwired: 3 in]
                n188 = local read "工位号"() -> (w978:enum16{"工位1", "工位2"})
                n189 = Set Menu Item Info(6:w973, 7:"USER_BLASTING_REC" ("项标识符"), 8:w971, 9:w973, 11:w972) -> (0:w967:errorcluster, 3:w968:refnum<k9>)  [unwired: 2 in]
                n190 = property on="工位号" class="Enum (严格)"("Val(Sgnl)"=w978) -> ()  [unwired: 2 in, 2 out]
                n191 = Set Menu Item Info(6:FALSE ("已勾选"), 7:"USER_BREATHE_REC" ("项标识符"), 8:w967, 9:TRUE ("已启用"), 11:w968) -> ()  [unwired: 2 in, 2 out]
              }
              frame "USER_BREATHE_REC" {
                w984 = TRUE ("已启用")
                n192 = Current VI's Menubar() -> (w991:refnum<k9>)
                n193 = Set Menu Item Info(6:FALSE ("已勾选"), 7:"USER_DATA_ALL" ("项标识符"), 9:TRUE ("已启用"), 11:w991) -> (0:w985:errorcluster, 3:w986:refnum<k9>)  [unwired: 3 in]
                n194 = local read "工位号"() -> (w992:enum16{"工位1", "工位2"})
                n195 = Set Menu Item Info(6:FALSE ("已勾选"), 7:"USER_BLASTING_REC" ("项标识符"), 8:w985, 9:TRUE ("已启用"), 11:w986) -> (0:w981:errorcluster, 3:w982:refnum<k9>)  [unwired: 2 in]
                n196 = property on="工位号" class="Enum (严格)"("Val(Sgnl)"=w992) -> ()  [unwired: 2 in, 2 out]
                n197 = Set Menu Item Info(6:w984, 7:"USER_BREATHE_REC" ("项标识符"), 8:w981, 9:w984, 11:w982) -> ()  [unwired: 2 in, 2 out]
              }
            }
          }
          event "确定按钮": Value Change {
            n198 = event-data() -> ()  [unwired: 1 in, 6 out]
            n199 = local read "PLC_Hd"() -> (w1000:refnum<class "Modbus Master.lvclass">)
            n200 = call "ConvertData.vi"("数组"="数组") -> ("数组 2"=w993:u16[])  [unwired: 10 in]
            n201 = call-dynamic "Write Single Holding Register.vi"("holding register value"="启动信号", "address"=u16 6000, "Modbus master in"=w1000) -> ("error out"=w998:errorcluster, "Modbus master out"=w999:refnum<class "Modbus Master.lvclass">)  [unwired: 7 in]
            n202 = call-dynamic "Write Multiple Holding Registers.vi"("error in (no error)"=w998, "holding register values"=w993, "starting address"=u16 6002 ("address"), "Modbus master in"=w999) -> ()  [unwired: 6 in, 2 out]
          }
          event "确定按钮 2": Value Change {
            n203 = event-data() -> ()  [unwired: 1 in, 6 out]
            n204 = local read "PLC_Hd"() -> (w1008:refnum<class "Modbus Master.lvclass">)
            n205 = call "ConvertData.vi"("数组"="数组 2") -> ("数组 2"=w1001:u16[])  [unwired: 10 in]
            n206 = call-dynamic "Write Single Holding Register.vi"("holding register value"="启动信号 2", "address"=u16 6100, "Modbus master in"=w1008) -> ("error out"=w1004:errorcluster, "Modbus master out"=w1005:refnum<class "Modbus Master.lvclass">)  [unwired: 7 in]
            n207 = call-dynamic "Write Multiple Holding Registers.vi"("error in (no error)"=w1004, "holding register values"=w1001, "starting address"=u16 6102 ("address"), "Modbus master in"=w1005) -> ()  [unwired: 6 in, 2 out]
          }
        }
        n208 = local read "bExit?"() -> (w584:bool)
        n209 = Or(x=w586, y=w584) -> (x .or. y?=w585:bool)
      }
      n210 = Current VI's Menubar() -> (w46:refnum<k9>)
      n211 = Greater Or Equal?(x=w44, y=2) -> (x >= y?=w40:bool)
      n212 = Set Menu Item Info(7:"USER_MANAGEMENT" ("项标识符"), 9:w40, 11:w46) -> (0:w43:errorcluster, 3:w35:refnum<k9>)  [unwired: 4 in]
      n213 = Select(t=T2."Enabled" ("禁用"), s=w40, f=T2."Disabled and Grayed Out" ("禁用")) -> (s? t:f=w37:T2)
      n214 = property on="Cpk保存路径" class="Path"(error in=w43, "DisabledEnum"=w37) -> (error out=w42:errorcluster)  [unwired: 1 in, 1 out]
      n215 = property on="Btn_保存报告" class="Bool"(error in=w42, "DisabledEnum"=w37) -> (error out=w36:errorcluster)  [unwired: 1 in, 1 out]
      n216 = Set Menu Item Info(7:"USER_DATANALYZE" ("项标识符"), 8:w36, 9:FALSE ("已启用"), 11:w35) -> ()  [unwired: 3 in, 2 out]
      n217 = call-poly <vilib>:"Create Master Instance.vi"("port (502)"=u16 502, "address"="192.168.10.100") -> ("error out"=w13:errorcluster, "TCP master instance"=w14:refnum<class "Modbus Master.lvclass">)  [unwired: 8 in]
      "PLC_Hd" <- w14
      n218 = while {
        shift-right: [w113] -> _
        shift-left: StationAction."Init" -> [w118]
        shift-right: [w111] -> _
        shift-left: string[][] [] ("工位1_数据表显示") -> [w112]
        shift-right: [w109] -> w22
        shift-left: "" -> [w110]
        shift-right: [w103] -> _
        shift-left: w27 -> [w107]
        shift-right: [w102] -> _
        shift-left: w27 -> [w106]
        shift-right: [w100] -> _
        shift-left: w27 -> [w105]
        shift-right: [w101] -> _
        shift-left: i32[] [] -> [w104]
        tunnel: u16 6100 ("starting address") -> [w99]
        tunnel: w13 -> [_]
        stop <- w117 stop-if-true
        n219 = local read "PLC_Hd"() -> (w98:refnum<class "Modbus Master.lvclass">)
        n220 = case shown="\"Done\"" w118 {
          tunnel: [_ _ _ TRUE] -> w117
          tunnel: [StationAction."Monitor" w162 StationAction."Monitor" StationAction."Exit"] -> w114
          tunnel: w98 -> [_ w134 w243 _]
          tunnel: w112 -> [_ w164 _ _]
          tunnel: [string[][] [] ("工位1_数据表显示") w163 string[][] [] ("工位1_数据表显示") string[][] [] ("工位1_数据表显示")] -> w111
          tunnel: w110 -> [w121 w161 w276 w337]
          tunnel: [w121 w160 "" w337] -> w109
          tunnel: [w120 w154 w316 w334] -> w103
          tunnel: [w120 w153 w316 w333] -> w102
          tunnel: [w120 w152 w316 w332] -> w100
          tunnel: [i32[] [] w155 i32[] [] w335] -> w101
          tunnel: w107 -> [_ w159 _ w334]
          tunnel: w106 -> [_ w158 _ w333]
          tunnel: w105 -> [_ w157 _ w332]
          tunnel: w104 -> [_ w156 _ w335]
          tunnel: w99 -> [_ w131 w242 _]
          frame "Init", Default {
            w120 = dbl[] []
          }
          frame "Monitor" {
            n221 = call-dynamic "Read Holding Registers.vi"("number of holding registers"=u16 80, "starting address"=w131, "Modbus master in"=w134) -> ("error out"=w137:errorcluster, "register values"=w136:u16[])  [unwired: 6 in, 1 out]
            n222 = Get Date/Time In Seconds() -> (seconds since 1Jan1904=w145:timestamp)
            n223 = call "解析寄电器.vi"("error in (no error)"=w137, "寄存器in"=w136) -> ("error out"=→"error out":errorcluster, "分解后报文out"=w133:string[], "原始报文out"=w132:string, "启动信号out"=w130:i32)  [unwired: 6 in]
            n224 = Index Array(array=w133, index #1=0 ("索引"), index #2=2 ("索引"), index #3=3 ("索引"), index #4=4 ("索引")) -> (element #2=w125:string, element #3=w138:string, element #4=w141:string)  [unwired: 1 out]
            n225 = Format Date/Time String(time format string (%c)="%H:%M:%S" ("时间格式字符串(%c)"), seconds (now)=w145) -> (date/time string=w148:string)  [unwired: 1 in]
            n226 = Format Date/Time String(time format string (%c)="%Y/%m/%d %H:%M:%S" ("时间格式字符串(%c)"), seconds (now)=w145) -> (date/time string=w144:string)  [unwired: 1 in]
            n227 = Decimal String To Number(string=w141) -> (number=w139:i32)  [unwired: 2 in, 1 out]
            n228 = Search and Replace String(replace all?=TRUE ("替换全部？(F)"), input string=w125, search string="\u0000" ("子字符串(\"\")"), replace string="") -> (result string=w124:string)  [unwired: 4 in, 3 out]
            n229 = local write "工位2_实时压力_Ind"(w138) -> ()
            n230 = case shown="1" w139 {
              tunnel: ["无效测试" "下呼吸测试" "上呼吸测试" "爆破测试"] -> w140
              frame 0, Default {
              }
              frame 1 {
              }
              frame 2 {
              }
              frame 3 {
              }
            }
            n231 = local write "工位2_产品型号"(w124) -> ()
            n232 = Build Array(w148, w138, w140) -> (w147:string[])
            n233 = Build Array (concatenate)(w164, w147) -> (w163:string[][])
            n234 = case shown="1" w130 {
              tunnel: [StationAction."Monitor" StationAction."Monitor" StationAction."Done"] -> w162
              tunnel: w161 -> [w182 w197 w236]
              tunnel: w144 -> [_ w199 _]
              tunnel: [w182 w198 w233] -> w160
              tunnel: w159 -> [w177 w196 w240]
              tunnel: w158 -> [w178 w195 w239]
              tunnel: w157 -> [w179 w194 w238]
              tunnel: w139 -> [_ w193 _]
              tunnel: [w181 w191 w237] -> w155
              tunnel: [w177 w190 w240] -> w154
              tunnel: [w178 w189 w239] -> w153
              tunnel: [w179 w188 w238] -> w152
              tunnel: w156 -> [w181 w192 w237]
              tunnel: w138 -> [_ w186 _]
              tunnel: w132 -> [_ _ w234]
              frame 0, Default {
              }
              frame 1 {
                n235 = Scan Value(string=w186, format string="%.3f" ("格式字符串")) -> (value=w185:dbl)  [unwired: 1 in, 1 out]
                n236 = Empty String/Path?(string/path=w197) -> (empty?=w183:bool)
                n237 = case shown="真" w183 {
                  frame False {
                  }
                  frame True {
                    n238 = local write "工位2_数据图表显示"(cluster{i32[], dbl[]}[] [] ("添加的数组")) -> ()
                  }
                }
                n239 = case shown="0, 默认" w193 {
                  tunnel: w196 -> [w208 w216 w224 w232]
                  tunnel: w195 -> [w207 w213 w222 w230]
                  tunnel: w194 -> [w206 w211 w220 w228]
                  tunnel: [w208 w214 w223 w231] -> w190
                  tunnel: [w207 w212 w221 w229] -> w189
                  tunnel: [w206 w209 w219 w227] -> w188
                  tunnel: w185 -> [_ w215 w218 w226]
                  tunnel: nan -> [_ w210 w217 w225]
                  frame 0, Default {
                  }
                  frame 1 {
                    n240 = Build Array (concatenate)(w213, w210) -> (w212:dbl[])
                    n241 = Build Array (concatenate)(w216, w215) -> (w214:dbl[])
                    n242 = Build Array (concatenate)(w211, w210) -> (w209:dbl[])
                  }
                  frame 2 {
                    n243 = Build Array (concatenate)(w222, w218) -> (w221:dbl[])
                    n244 = Build Array (concatenate)(w224, w217) -> (w223:dbl[])
                    n245 = Build Array (concatenate)(w220, w217) -> (w219:dbl[])
                  }
                  frame 3 {
                    n246 = Build Array (concatenate)(w230, w225) -> (w229:dbl[])
                    n247 = Build Array (concatenate)(w232, w225) -> (w231:dbl[])
                    n248 = Build Array (concatenate)(w228, w226) -> (w227:dbl[])
                  }
                }
                n249 = case shown="1, 默认" w193 {
                  tunnel: w192 -> [w202 w204]
                  tunnel: [w202 w203] -> w191
                  frame 0 {
                  }
                  frame 1, Default {
                    n250 = Array Size(array=w204) -> (size(s)=w205:i32)
                    n251 = Build Array (concatenate)(w204, w205) -> (w203:i32[])
                  }
                }
                n252 = Select(t=w199, s=w183, f=w197) -> (s? t:f=w198:string)
              }
              frame 2 {
                n253 = Concatenate Strings(w236, "|", w234) -> (w233:string)
              }
            }
            n254 = case shown="1, 默认" w130 {
              tunnel: w155 -> [_ w172]
              tunnel: w154 -> [_ w171]
              tunnel: w153 -> [_ w170]
              tunnel: w152 -> [_ w169]
              frame 0 {
              }
              frame 1, Default {
                n255 = Bundle(w172, w171) -> (w166:cluster{i32[], dbl[]})  [unwired: 1 in]
                n256 = Bundle(w172, w170) -> (w167:cluster{i32[], dbl[]})  [unwired: 1 in]
                n257 = Bundle(w172, w169) -> (w168:cluster{i32[], dbl[]})  [unwired: 1 in]
                n258 = Build Array(w166, w167, w168) -> (w165:cluster{i32[], dbl[]}[])
                n259 = local write "工位2_数据图表显示"(w165) -> ()
              }
            }
          }
          frame "Done" {
            w250 = FALSE ("CloseFPAfterCall")
            w280 = TRUE ("忽略大小写？(F)")
            w278 = ""
            w316 = dbl[] []
            n260 = for {
              N: 3 -> [_]
              tunnel: w242 -> [w323]
              shift-right: [w322] -> _
              shift-left: w243 -> [w330]
              stop <- w320 stop-if-true
              n261 = call-dynamic "Write Single Holding Register.vi"("holding register value"=u16 0 ("address"), "address"=w323, "Modbus master in"=w330) -> ("error out"=w325:errorcluster, "Modbus master out"=w324:refnum<class "Modbus Master.lvclass">)  [unwired: 7 in]
              n262 = call-dynamic "Read Holding Registers.vi"("error in (no error)"=w325, "number of holding registers"=u16 80, "starting address"=w323, "Modbus master in"=w324) -> ("error out"=w327:errorcluster, "register values"=w328:u16[], "Modbus master out"=w322:refnum<class "Modbus Master.lvclass">)  [unwired: 5 in]
              n263 = call "解析寄电器.vi"("error in (no error)"=w327, "寄存器in"=w328) -> ("启动信号out"=w321:i32)  [unwired: 6 in, 3 out]
              n264 = Equal To 0?(x=w321) -> (x = 0?=w320:bool)
              n265 = case shown="假" w320 {
                frame False {
                  n266 = Wait Until Next ms Multiple(millisecond multiple=u32 1000 ("毫秒倍数")) -> ()  [unwired: 1 out]
                }
                frame True {
                }
              }
            }
            n267 = Get Date/Time In Seconds() -> (seconds since 1Jan1904=w273:timestamp)
            n268 = Format Date/Time String(time format string (%c)="%Y/%m/%d %H:%M:%S" ("时间格式字符串(%c)"), seconds (now)=w273) -> (date/time string=w290:string)  [unwired: 1 in]
            n269 = Match Pattern(string=w276, regular expression="|") -> (before substring=w306:string, after substring=w305:string)  [unwired: 1 in, 2 out]
            n270 = call "检查并创建文件夹.vi"("路径in"=path "D:/气压数据记录文件/工位2/气压数据记录.csv") -> ("error out"=w302:errorcluster, "dup path"=w303:path)  [unwired: 9 in]
            n271 = Format Into String(format string="%s;%s;%s\n" ("格式字符串"), w306, w290, w305) -> (resulting string=w284:string)  [unwired: 2 in, 1 out]
            n272 = call "打开数据记录文件.vi"("错误输入"=w302, "路径in"=w303) -> ("error out"=w300:errorcluster, "引用句柄输出"=w301:refnum<file>)  [unwired: 8 in]
            n273 = Search and Replace String(case sensitive?=w280, input string=w284, search string="\n\r", replace string=w278) -> (result string=w281:string)  [unwired: 4 in, 3 out]
            n274 = Set File Position(refnum=w301, from (0:start)=enum16{"start", "end", "current"}."end" ("自（0:起始）"), error in=w300) -> (refnum out=w313:refnum<file>, error out=w311:errorcluster)  [unwired: 1 in]
            n275 = Format Date/Time String(time format string (%c)="%Y-%m-%d_%H-%M-%S" ("时间格式字符串(%c)"), seconds (now)=w273) -> (date/time string=w275:string)  [unwired: 1 in]
            n276 = Search and Replace String(replace all?=w280, input string=w281, search string="\u0000", replace string=w278) -> (result string=w277:string)  [unwired: 4 in, 3 out]
            n277 = Spreadsheet String To Array(delimiter (Tab)=";" ("分隔符(Tab)"), format string="%s" ("格式字符串"), spreadsheet string=w277, array type (2D Dbl)=string[] []) -> (array=w283:string[])
            n278 = Write to Text File(file (use dialog)=w313, text=w284, error in=w311) -> (refnum out=w309:refnum<file>, error out=w310:errorcluster)  [unwired: 1 in, 1 out]
            n279 = Close File(refnum=w309, error in=w310) -> ()  [unwired: 2 out]
            n280 = Index Array(array=w283, index #1=4 ("索引"), index #2=6 ("索引"), index #3=21 ("索引")) -> (element #1=w295:string, element #2=w292:string, element #3=w291:string)
            n281 = Format Into String(format string="%s-%s-%s-%s.xlsx" ("格式字符串"), w295, w292, w291, w275) -> (resulting string=w288:string)  [unwired: 2 in, 1 out]
            n282 = call <vilib>:"Application Directory.vi"() -> ("Application Directory"=w257:path)
            n283 = Build Path(base path=path "D:/报告文件/工位2" ("路径in"), name or relative path=w288) -> (appended path=w287:path)
            n284 = Build Path(base path=w257, name or relative path="SubVIs\\GeneratorTestReport.vi" ("viPath")) -> (appended path=w256:path)
            n285 = local read "工位2_数据图表显示"() -> (w286:cluster{i32[], dbl[]}[])
            n286 = Path To String(path=w256) -> (string=w255:string)
            n287 = Automation Open(Automation Refnum="LabVIEW._Application 5", 9:TRUE ("open new instance (false)")) -> (Automation Refnum=w265:refnum<k7>, error out=w264:errorcluster)  [unwired: 2 in]
            n288 = invoke class="_Application" method="GetVIReference"(reference=w265, error in=w264, "viPath"=w255, "resvForCall"=FALSE, "options"=0) -> (reference out=w258:refnum<k7>, error out=w262:errorcluster, "GetVIReference"=w263:refnum<k7>)  [unwired: 2 in, 4 out]
            n289 = To Variant(anything=w286) -> (Variant=w268:variant)
            n290 = To Variant(anything=w284) -> (Variant=w269:variant)
            n291 = To Variant(anything=errorcluster {"status"=FALSE, "code"=0, "source"=""} ("错误输出")) -> (Variant=w270:variant)
            n292 = To Variant(anything=errorcluster {"status"=FALSE, "code"=0, "source"=""} ("错误输出")) -> (Variant=w272:variant)
            n293 = To Variant(anything=w287) -> (Variant=w267:variant)
            n294 = Build Array(w267, w268, w269, w270, w272) -> (w271:variant[])
            n295 = invoke class="VirtualInstrument" method="Call2"(reference=w263, error in=w262, "paramNames"=string[] ["路径in", "图表数据in", "Record in", "error in (no error)", "error out"], "paramVals"=w271, "openFP"=w250, "CloseFPAfterCall"=TRUE, "SuspendOnCall"=w250) -> (reference out=w261:refnum<k7>, error out=w260:errorcluster, "paramVals"=w245:variant)  [unwired: 2 in, 6 out]
            n296 = local write "paramVals"(w245) -> ()
            n297 = Close Reference(reference=w261, error in (no error)=w260) -> (error out=w259:errorcluster)
            n298 = Close Reference(reference=w258, error in (no error)=w259) -> ()  [unwired: 1 out]
          }
          frame "Exit" {
          }
        }
        n299 = local read "bExit?"() -> (w116:bool)
        n300 = Select(t=StationAction."Exit", s=w116, f=w114) -> (s? t:f=w113:T1)
        n301 = Wait Until Next ms Multiple(millisecond multiple=u32 50 ("毫秒倍数")) -> ()  [unwired: 1 out]
      }
      n302 = while {
        shift-right: [w355] -> _
        shift-left: StationAction."Init" -> [w360]
        shift-right: [w353] -> _
        shift-left: string[][] [] ("工位1_数据表显示") -> [w354]
        shift-right: [w351] -> w15
        shift-left: "" -> [w352]
        shift-right: [w345] -> _
        shift-left: w28 -> [w349]
        shift-right: [w344] -> _
        shift-left: w28 -> [w348]
        shift-right: [w342] -> _
        shift-left: w28 -> [w347]
        shift-right: [w343] -> _
        shift-left: i32[] [] -> [w346]
        tunnel: u16 6000 ("starting address") -> [w341]
        tunnel: w13 -> [_]
        stop <- w359 stop-if-true
        n303 = local read "PLC_Hd"() -> (w340:refnum<class "Modbus Master.lvclass">)
        n304 = case shown="\"Done\"" w360 {
          tunnel: [_ _ _ TRUE] -> w359
          tunnel: [StationAction."Monitor" w404 StationAction."Monitor" StationAction."Exit"] -> w356
          tunnel: w340 -> [_ w393 w525 _]
          tunnel: w354 -> [_ w406 _ _]
          tunnel: [string[][] [] ("工位1_数据表显示") w405 string[][] [] ("工位1_数据表显示") string[][] [] ("工位1_数据表显示")] -> w353
          tunnel: w352 -> [w363 w403 w516 w579]
          tunnel: [w363 w402 "" w579] -> w351
          tunnel: [w362 w396 w558 w576] -> w345
          tunnel: [w362 w395 w558 w575] -> w344
          tunnel: [w362 w394 w558 w574] -> w342
          tunnel: [i32[] [] w397 i32[] [] w577] -> w343
          tunnel: w349 -> [_ w401 _ w576]
          tunnel: w348 -> [_ w400 _ w575]
          tunnel: w347 -> [_ w399 _ w574]
          tunnel: w346 -> [_ w398 _ w577]
          tunnel: w341 -> [_ w373 w524 _]
          frame "Init", Default {
            w362 = dbl[] []
          }
          frame "Monitor" {
            n305 = call-dynamic "Read Holding Registers.vi"("number of holding registers"=u16 80, "starting address"=w373, "Modbus master in"=w393) -> ("error out"=w377:errorcluster, "register values"=w376:u16[])  [unwired: 6 in, 1 out]
            n306 = Get Date/Time In Seconds() -> (seconds since 1Jan1904=w386:timestamp)
            n307 = call "解析寄电器.vi"("error in (no error)"=w377, "寄存器in"=w376) -> ("error out"=→"error out 2":errorcluster, "分解后报文out"=w375:string[], "原始报文out"=w374:string, "启动信号out"=w372:i32)  [unwired: 6 in]
            n308 = Index Array(array=w375, index #1=0 ("索引"), index #2=2 ("索引"), index #3=3 ("索引"), index #4=4 ("索引")) -> (element #2=w370:string, element #3=w379:string, element #4=w382:string)  [unwired: 1 out]
            n309 = Format Date/Time String(time format string (%c)="%H:%M:%S" ("时间格式字符串(%c)"), seconds (now)=w386) -> (date/time string=w389:string)  [unwired: 1 in]
            n310 = Format Date/Time String(time format string (%c)="%Y/%m/%d %H:%M:%S" ("时间格式字符串(%c)"), seconds (now)=w386) -> (date/time string=w385:string)  [unwired: 1 in]
            n311 = Decimal String To Number(string=w382) -> (number=w380:i32)  [unwired: 2 in, 1 out]
            n312 = Search and Replace String(replace all?=TRUE ("替换全部？(F)"), input string=w370, search string="\u0000" ("子字符串(\"\")"), replace string="") -> (result string=w367:string)  [unwired: 4 in, 3 out]
            n313 = local write "工位1_产品型号"(w367) -> ()
            n314 = local write "工位1_实时压力_Ind"(w379) -> ()
            n315 = case shown="1" w380 {
              tunnel: ["无效测试" "下呼吸测试" "上呼吸测试" "爆破测试"] -> w381
              frame 0, Default {
              }
              frame 1 {
              }
              frame 2 {
              }
              frame 3 {
              }
            }
            n316 = Build Array(w389, w379, w381) -> (w388:string[])
            n317 = Build Array (concatenate)(w406, w388) -> (w405:string[][])
            n318 = local write "工位1_数据表显示"(w405) -> ()
            n319 = case shown="1" w372 {
              tunnel: [StationAction."Monitor" StationAction."Monitor" StationAction."Done"] -> w404
              tunnel: w403 -> [w424 w439 w478]
              tunnel: w385 -> [_ w441 _]
              tunnel: [w424 w440 w475] -> w402
              tunnel: w401 -> [w422 w438 w482]
              tunnel: w400 -> [w421 w437 w481]
              tunnel: w399 -> [w420 w436 w480]
              tunnel: w380 -> [_ w435 _]
              tunnel: [w423 w433 w479] -> w397
              tunnel: [w422 w432 w482] -> w396
              tunnel: [w421 w431 w481] -> w395
              tunnel: [w420 w430 w480] -> w394
              tunnel: w398 -> [w423 w434 w479]
              tunnel: w379 -> [_ w428 _]
              tunnel: w374 -> [_ _ w476]
              frame 0, Default {
              }
              frame 1 {
                n320 = Empty String/Path?(string/path=w439) -> (empty?=w425:bool)
                n321 = case shown="真" w425 {
                  frame False {
                  }
                  frame True {
                    n322 = local write "工位1_数据图表显示"(cluster{i32[], dbl[]}[] [] ("添加的数组")) -> ()
                  }
                }
                n323 = Scan Value(string=w428, format string="%.3f" ("格式字符串")) -> (value=w427:dbl)  [unwired: 1 in, 1 out]
                n324 = case shown="0, 默认" w435 {
                  tunnel: w438 -> [w450 w458 w466 w474]
                  tunnel: w437 -> [w449 w455 w464 w472]
                  tunnel: w436 -> [w448 w453 w462 w470]
                  tunnel: [w450 w456 w465 w473] -> w432
                  tunnel: [w449 w454 w463 w471] -> w431
                  tunnel: [w448 w451 w461 w469] -> w430
                  tunnel: w427 -> [_ w457 w460 w468]
                  tunnel: nan -> [_ w452 w459 w467]
                  frame 0, Default {
                  }
                  frame 1 {
                    n325 = Build Array (concatenate)(w455, w452) -> (w454:dbl[])
                    n326 = Build Array (concatenate)(w458, w457) -> (w456:dbl[])
                    n327 = Build Array (concatenate)(w453, w452) -> (w451:dbl[])
                  }
                  frame 2 {
                    n328 = Build Array (concatenate)(w464, w460) -> (w463:dbl[])
                    n329 = Build Array (concatenate)(w466, w459) -> (w465:dbl[])
                    n330 = Build Array (concatenate)(w462, w459) -> (w461:dbl[])
                  }
                  frame 3 {
                    n331 = Build Array (concatenate)(w472, w467) -> (w471:dbl[])
                    n332 = Build Array (concatenate)(w474, w467) -> (w473:dbl[])
                    n333 = Build Array (concatenate)(w470, w468) -> (w469:dbl[])
                  }
                }
                n334 = case shown="1, 默认" w435 {
                  tunnel: w434 -> [w444 w446]
                  tunnel: [w444 w445] -> w433
                  frame 0 {
                  }
                  frame 1, Default {
                    n335 = Array Size(array=w446) -> (size(s)=w447:i32)
                    n336 = Build Array (concatenate)(w446, w447) -> (w445:i32[])
                  }
                }
                n337 = Select(t=w441, s=w425, f=w439) -> (s? t:f=w440:string)
              }
              frame 2 {
                n338 = Concatenate Strings(w478, "|", w476) -> (w475:string)
              }
            }
            n339 = case shown="1, 默认" w372 {
              tunnel: w397 -> [_ w414]
              tunnel: w396 -> [_ w413]
              tunnel: w395 -> [_ w412]
              tunnel: w394 -> [_ w411]
              frame 0 {
              }
              frame 1, Default {
                n340 = Bundle(w414, w413) -> (w407:cluster{i32[], dbl[]})  [unwired: 1 in]
                n341 = Bundle(w414, w412) -> (w408:cluster{i32[], dbl[]})  [unwired: 1 in]
                n342 = Bundle(w414, w411) -> (w409:cluster{i32[], dbl[]})  [unwired: 1 in]
                n343 = Build Array(w407, w408, w409) -> (w410:cluster{i32[], dbl[]}[])
                n344 = local write "工位1_数据图表显示"(w410) -> ()
              }
            }
          }
          frame "Done" {
            w489 = FALSE ("CloseFPAfterCall")
            w519 = TRUE ("忽略大小写？(F)")
            w517 = ""
            w558 = dbl[] []
            n345 = for {
              N: 3 -> [_]
              tunnel: w524 -> [w565]
              shift-right: [w564] -> _
              shift-left: w525 -> [w572]
              stop <- w562 stop-if-true
              n346 = call-dynamic "Write Single Holding Register.vi"("holding register value"=u16 0 ("address"), "address"=w565, "Modbus master in"=w572) -> ("error out"=w567:errorcluster, "Modbus master out"=w566:refnum<class "Modbus Master.lvclass">)  [unwired: 7 in]
              n347 = call-dynamic "Read Holding Registers.vi"("error in (no error)"=w567, "number of holding registers"=u16 80, "starting address"=w565, "Modbus master in"=w566) -> ("error out"=w569:errorcluster, "register values"=w570:u16[], "Modbus master out"=w564:refnum<class "Modbus Master.lvclass">)  [unwired: 5 in]
              n348 = call "解析寄电器.vi"("error in (no error)"=w569, "寄存器in"=w570) -> ("启动信号out"=w563:i32)  [unwired: 6 in, 3 out]
              n349 = Equal To 0?(x=w563) -> (x = 0?=w562:bool)
              n350 = case shown="假" w562 {
                frame False {
                  n351 = Wait Until Next ms Multiple(millisecond multiple=u32 1000 ("毫秒倍数")) -> ()  [unwired: 1 out]
                }
                frame True {
                }
              }
            }
            n352 = Get Date/Time In Seconds() -> (seconds since 1Jan1904=w514:timestamp)
            n353 = Format Date/Time String(time format string (%c)="%Y/%m/%d %H:%M:%S" ("时间格式字符串(%c)"), seconds (now)=w514) -> (date/time string=w529:string)  [unwired: 1 in]
            n354 = Match Pattern(string=w516, regular expression="|") -> (before substring=w548:string, after substring=w547:string)  [unwired: 1 in, 2 out]
            n355 = Format Into String(format string="%s;%s;%s\n" ("格式字符串"), w548, w529, w547) -> (resulting string=w523:string)  [unwired: 2 in, 1 out]
            n356 = Format Date/Time String(time format string (%c)="%Y-%m-%d_%H-%M-%S" ("时间格式字符串(%c)"), seconds (now)=w514) -> (date/time string=w513:string)  [unwired: 1 in]
            n357 = call "检查并创建文件夹.vi"("路径in"=path "D:/气压数据记录文件/工位1/气压数据记录.csv") -> ("error out"=w544:errorcluster, "dup path"=w545:path)  [unwired: 9 in]
            n358 = Search and Replace String(case sensitive?=w519, input string=w523, search string="\n\r", replace string=w517) -> (result string=w521:string)  [unwired: 4 in, 3 out]
            n359 = Search and Replace String(replace all?=w519, input string=w521, search string="\u0000", replace string=w517) -> (result string=w520:string)  [unwired: 4 in, 3 out]
            n360 = call "打开数据记录文件.vi"("错误输入"=w544, "路径in"=w545) -> ("error out"=w542:errorcluster, "引用句柄输出"=w543:refnum<file>)  [unwired: 8 in]
            n361 = Set File Position(refnum=w543, from (0:start)=enum16{"start", "end", "current"}."end" ("自（0:起始）"), error in=w542) -> (refnum out=w555:refnum<file>, error out=w553:errorcluster)  [unwired: 1 in]
            n362 = Spreadsheet String To Array(delimiter (Tab)=";" ("分隔符(Tab)"), format string="%s" ("格式字符串"), spreadsheet string=w520, array type (2D Dbl)=string[] []) -> (array=w537:string[])
            n363 = Write to Text File(file (use dialog)=w555, text=w523, error in=w553) -> (refnum out=w551:refnum<file>, error out=w552:errorcluster)  [unwired: 1 in, 1 out]
            n364 = call <vilib>:"Application Directory.vi"() -> ("Application Directory"=w496:path)
            n365 = Close File(refnum=w551, error in=w552) -> ()  [unwired: 2 out]
            n366 = Index Array(array=w537, index #1=4 ("索引"), index #2=6 ("索引"), index #3=21 ("索引")) -> (element #1=w534:string, element #2=w531:string, element #3=w530:string)
            n367 = Build Path(base path=w496, name or relative path="SubVIs\\GeneratorTestReport.vi" ("viPath")) -> (appended path=w495:path)
            n368 = Format Into String(format string="%s-%s-%s-%s.xlsx" ("格式字符串"), w534, w531, w530, w513) -> (resulting string=w527:string)  [unwired: 2 in, 1 out]
            n369 = Path To String(path=w495) -> (string=w494:string)
            n370 = Automation Open(Automation Refnum="LabVIEW._Application 4", 9:TRUE ("open new instance (false)")) -> (Automation Refnum=w504:refnum<k7>, error out=w503:errorcluster)  [unwired: 2 in]
            n371 = local read "工位1_数据图表显示"() -> (w541:cluster{i32[], dbl[]}[])
            n372 = Build Path(base path=path "D:/报告文件/工位1" ("路径in"), name or relative path=w527) -> (appended path=w526:path)
            n373 = invoke class="_Application" method="GetVIReference"(reference=w504, error in=w503, "viPath"=w494, "resvForCall"=FALSE, "options"=0) -> (reference out=w497:refnum<k7>, error out=w501:errorcluster, "GetVIReference"=w502:refnum<k7>)  [unwired: 2 in, 4 out]
            n374 = To Variant(anything=w526) -> (Variant=w506:variant)
            n375 = To Variant(anything=w541) -> (Variant=w507:variant)
            n376 = To Variant(anything=w523) -> (Variant=w508:variant)
            n377 = To Variant(anything=errorcluster {"status"=FALSE, "code"=0, "source"=""} ("错误输出")) -> (Variant=w509:variant)
            n378 = To Variant(anything=errorcluster {"status"=FALSE, "code"=0, "source"=""} ("错误输出")) -> (Variant=w512:variant)
            n379 = Build Array(w506, w507, w508, w509, w512) -> (w510:variant[])
            n380 = invoke class="VirtualInstrument" method="Call2"(reference=w502, error in=w501, "paramNames"=string[] ["路径in", "图表数据in", "Record in", "error in (no error)", "error out"], "paramVals"=w510, "openFP"=w489, "CloseFPAfterCall"=TRUE, "SuspendOnCall"=w489) -> (reference out=w500:refnum<k7>, error out=w499:errorcluster, "paramVals"=→"paramVals":variant)  [unwired: 2 in, 6 out]
            n381 = Close Reference(reference=w500, error in (no error)=w499) -> (error out=w498:errorcluster)
            n382 = Close Reference(reference=w497, error in (no error)=w498) -> ()  [unwired: 1 out]
          }
          frame "Exit" {
          }
        }
        n383 = local read "bExit?"() -> (w358:bool)
        n384 = Select(t=StationAction."Exit", s=w358, f=w356) -> (s? t:f=w355:T1)
        n385 = Wait Until Next ms Multiple(millisecond multiple=u32 50 ("毫秒倍数")) -> ()  [unwired: 1 out]
      }
      n386 = while {
        shift-right: [w54] -> w16
        shift-left: w14 -> [w64]
        tunnel: u16 6300 ("starting address") -> [w53]
        tunnel: w13 -> [w52]
        stop <- w49 stop-if-true
        n387 = call-dynamic "Read Holding Registers.vi"("error in (no error)"=w52, "number of holding registers"=u16 1, "starting address"=w53, "Modbus master in"=w64) -> ("error out"=w51:errorcluster, "register values"=w62:u16[], "Modbus master out"=w57:refnum<class "Modbus Master.lvclass">)  [unwired: 5 in]
        n388 = Index Array(array=w62) -> (element=w61:u16)  [unwired: 1 in]
        n389 = Wait Until Next ms Multiple(millisecond multiple=u32 1000 ("毫秒倍数")) -> ()  [unwired: 1 out]
        n390 = Equal?(x=u16 2 ("starting address"), y=w61) -> (x = y?=w59:bool)
        n391 = case shown="真" w59 {
          tunnel: w57 -> [w72 w97]
          tunnel: [w71 w97] -> w55
          tunnel: w51 -> [w70 w96]
          tunnel: [w69 w96] -> w50
          tunnel: [w66 _] -> w48
          frame False {
            n392 = stacked-sequence {
              seq-local: [w73 _] -> [_ w78]
              tunnel: w72 -> [_ w82]
              tunnel: [_ w81] -> w71
              tunnel: w70 -> [_ w80]
              tunnel: [_ w79] -> w69
              tunnel: [w73 _] -> w66
              frame #0 {
                n393 = Two Button Dialog(message="PLC通讯失败，请先确认PLC是否已经连接，确认连接后点击“确认”按钮继续，如果关闭程序请点击“退出”按钮" ("消息"), 1:"退出" ("按钮名称（“确定”）"), 2:"确认" ("按钮名称（“确定”）")) -> (T button?=w74:bool)
                n394 = Not(x=w74) -> (.not. x?=w73:bool)
                n395 = local write "bExit?"(w73) -> ()
              }
              frame #1 {
                n396 = case shown="真" w78 {
                  tunnel: w82 -> [w91 w93]
                  tunnel: [w88 w93] -> w81
                  tunnel: w80 -> [w87 w92]
                  tunnel: [w85 w92] -> w79
                  frame False {
                    n397 = call <vilib>:"Clear Errors.vi"("error in (no error)"=w87) -> ("error out"=w86:errorcluster)  [unwired: 5 in, 1 out]
                    n398 = call-dynamic "Close.vi"("error in (no error)"=w86, "Modbus master in"=w91) -> ("error out"=w84:errorcluster)  [unwired: 9 in]
                    n399 = call <vilib>:"Clear Errors.vi"("error in (no error)"=w84) -> ("error out"=w83:errorcluster)  [unwired: 5 in, 1 out]
                    n400 = call-poly <vilib>:"Create Master Instance.vi"("error in (no error)"=w83, "port (502)"=u16 502, "address"="192.168.10.100") -> ("error out"=w85:errorcluster, "TCP master instance"=w88:refnum<class "Modbus Master.lvclass">)  [unwired: 7 in]
                  }
                  frame True {
                  }
                }
              }
            }
            n401 = property on="PLC状态显示" class="Str"("Value"="PLC连接异常" ("消息"), "Text.FG Color"=u32 16711680 ("文本.颜色:背景色")) -> ()  [unwired: 2 in, 2 out]
          }
          frame True {
            n402 = property on="PLC状态显示" class="Str"("Value"="PLC连接正常" ("消息"), "Text.FG Color"=u32 6618880 ("文本.颜色:背景色")) -> ()  [unwired: 2 in, 2 out]
          }
        }
        n403 = local read "bExit?"() -> (w63:bool)
        n404 = Or(x=w48, y=w63) -> (x .or. y?=w49:bool)
        n405 = call-dynamic "Write Single Holding Register.vi"("error in (no error)"=w50, "holding register value"=u16 1 ("address"), "address"=w53, "Modbus master in"=w55) -> ("error out"=→"error out 3":errorcluster, "Modbus master out"=w54:refnum<class "Modbus Master.lvclass">)  [unwired: 6 in]
        n406 = local write "PLC_Hd"(w54) -> ()
      }
      n407 = flat-sequence {
        tunnel: w22 -> [_]
        tunnel: w16 -> [w583]
        tunnel: w15 -> [_]
        frame #0 {
          n408 = call-dynamic "Close.vi"("Modbus master in"=w583) -> ("error out"=w582:errorcluster)  [unwired: 10 in]
          n409 = call <vilib>:"Clear Errors.vi"("error in (no error)"=w582) -> ()  [unwired: 5 in, 2 out]
        }
      }
    }
    frame True {
    }
  }
  "bExit?" <- FALSE ("bExit?")
  "工位1_数据表显示" <- string[][] [] ("工位1_数据表显示")
  "工位1_产品型号" <- w6
  "工位1_实时压力_Ind" <- w6
  "工位1_数据图表显示" <- w8
  "表格控件" <- w1
  "Cpk原始数据" <- w1
  "工位2_产品型号" <- w6
  "工位2_实时压力_Ind" <- w6
  "工位2_数据图表显示" <- w8
  "PLC状态显示" <- w6
  "原始表格" <- w1
